vi "ziExample-HF2-QControl.vi"() -> ()   [LabVIEW 2009]
doc: "Control a Zurich instrument device via the LabOne Labview API. \nRequirements: Zurich Instruments HF2LI with HF2-MF and HF2-PID options.\nThis LabVIEW vi helps in configuring an HF2 to do Q-Control.\n\n© Zurich Instruments AG, www.zhinst.com"
uses:
  <instrlib>/Zurich Instruments LabOne/Public/Configure/ziSetValueDouble.vi
  <vilib>/Analysis/NI_AALPro.lvlib
  <vilib>/Utility/NIReport.llb/NI_report.lvclass
  <instrlib>/Zurich Instruments LabOne/Zurich Instruments LabOne.lvlib
panel:
  in  "restore settings":bool caption="Restore original settings"
  out "fmax":dbl=1000.0
  out "fmin":dbl=1000.0
  in  "Tab Control Sweep":enum32{"Sweeper", "Advanced Settings", "Help"}(tab)
  in  "Drive (V)":dbl=0.01 format="%.3g"
  out "Resonance Frequency Q":dbl
  in  "Run":bool caption="Run Sweep"
  out "Sweep Progress":dbl(slide) max=21.0 scale=0.0..1.0
  out "Graph Phase":T1(graph)=[{"Output (F,X1,Y1,X2,Y2,...,Vo)"=[1841839.1959798995, 1841849.2462311557, 1841859.2964824121, 1841869.3467336684, 1841879.3969849246, 1841889.447236181, 1841899.4974874372, 1841909.5477386934, 1841919.5979899496, 1841929.648241206, 1841939.6984924623, 1841949.7487437185, 1841959.798994975, 1841969.8492462311, 1841979.8994974873, 1841989.9497487438, 1842000.0, 1842010.0502512562, 1842020.1005025127, 1842030.1507537689, 1842040.201005025, 1842050.2512562815, 1842060.3015075377, 1842070.351758794, 1842080.4020100501, 1842090.4522613066, 1842100.5025125628, 1842110.552763819, 1842120.6030150754, 1842130.6532663316, 1842140.7035175879, 1842150.7537688443, 1842160.8040201005, 1842170.8542713567, 1842180.9045226132, 1842190.9547738694, 1842201.0050251256, 1842211.055276382, 1842221.1055276382, 1842231.1557788944, 1842241.2060301506, 1842251.256281407, 1842261.3065326633, 1842271.3567839195, 1842281.407035176, 1842291.4572864322, 1842301.5075376884, 1842311.5577889448, 1842321.608040201, 1842331.6582914572, 1842341.7085427137, 1842351.7587939699, 1842361.809045226, 1842371.8592964825, 1842381.9095477387, 1842391.959798995, 1842402.0100502511, 1842412.0603015076, 1842422.1105527638, 1842432.16080402, 1842442.2110552764, 1842452.2613065327, 1842462.3115577889, 1842472.3618090453, 1842482.4120603015, 1842492.4623115577, 1842502.5125628142, 1842512.5628140704, 1842522.6130653266, 1842532.6633165828, 1842542.7135678392, 1842552.7638190954, 1842562.8140703517, 1842572.864321608, 1842582.9145728643, 1842592.9648241205, 1842603.015075377, 1842613.0653266332, 1842623.1155778894, 1842633.1658291458, 1842643.216080402, 1842653.2663316582, 1842663.3165829147, 1842673.3668341709, 1842683.417085427, 1842693.4673366833, 1842703.5175879397, 1842713.567839196, 1842723.6180904522, 1842733.6683417086, 1842743.7185929648, 1842753.768844221, 1842763.8190954775, 1842773.8693467337, 1842783.9195979899, 1842793.9698492463, 1842804.0201005025, 1842814.0703517587, 1842824.1206030152, 1842834.1708542714, 1842844.2211055276, 1842854.2713567838, 1842864.3216080402, 1842874.3718592965, 1842884.4221105527, 1842894.472361809, 1842904.5226130653, 1842914.5728643215, 1842924.623115578, 1842934.6733668342, 1842944.7236180904, 1842954.7738693468, 1842964.824120603, 1842974.8743718592, 1842984.9246231157, 1842994.974874372, 1843005.025125628, 1843015.0753768843, 1843025.1256281408, 1843035.175879397, 1843045.2261306532, 1843055.2763819096, 1843065.3266331658, 1843075.376884422, 1843085.4271356785, 1843095.4773869347, 1843105.527638191, 1843115.5778894473, 1843125.6281407035, 1843135.6783919598, 1843145.7286432162, 1843155.7788944724, 1843165.8291457286, 1843175.8793969848, 1843185.9296482413, 1843195.9798994975, 1843206.0301507537, 1843216.0804020101, 1843226.1306532663, 1843236.1809045225, 1843246.231155779, 1843256.2814070352, 1843266.3316582914, 1843276.3819095478, 1843286.432160804, 1843296.4824120603, 1843306.5326633165, 1843316.582914573, 1843326.6331658291, 1843336.6834170853, 1843346.7336683418, 1843356.783919598, 1843366.8341708542, 1843376.8844221106, 1843386.9346733668, 1843396.984924623, 1843407.0351758795, 1843417.0854271357, 1843427.135678392, 1843437.1859296483, 1843447.2361809046, 1843457.2864321608, 1843467.336683417, 1843477.3869346734, 1843487.4371859296, 1843497.4874371858, 1843507.5376884423, 1843517.5879396985, 1843527.6381909547, 1843537.6884422111, 1843547.7386934673, 1843557.7889447236, 1843567.83919598, 1843577.8894472362, 1843587.9396984924, 1843597.9899497489, 1843608.040201005, 1843618.0904522613, 1843628.1407035175, 1843638.190954774, 1843648.2412060301, 1843658.2914572863, 1843668.3417085428, 1843678.391959799, 1843688.4422110552, 1843698.4924623116, 1843708.5427135678, 1843718.592964824, 1843728.6432160805, 1843738.6934673367, 1843748.743718593, 1843758.7939698494, 1843768.8442211056, 1843778.8944723618, 1843788.944723618, 1843798.9949748744, 1843809.0452261306, 1843819.0954773868, 1843829.1457286433, 1843839.1959798995], "dX/dt"=[-6.94293659208085, -7.039263365714603, -7.015747865746605, -7.022831577183382, -7.070140649231355, -7.097687461922305, -7.105617775743133, -7.187018771027357, -7.215555605807255, -7.209120372797453, -7.222963353111247, -7.2482145424437725, -7.336471988299522, -7.392871009974112, -7.404378015656745, -7.392520359287413, -7.520355608686046, -7.519542598388936, -7.550628880706965, -7.581504623203495, -7.613602056591421, -7.5885724211422065, -7.700014320037284, -7.728140979121345, -7.810709171761543, -7.784263466588973, -7.881518062030821, -7.903674328964446, -7.971719351332499, -8.017529667992314, -8.058121436672986, -8.165785698106287, -8.19016022550502, -8.212700433959935, -8.32675261509468, -8.371215456694097, -8.455244319826404, -8.452589972505562, -8.593897328803308, -8.603598584374405, -8.66788383890823, -8.728838589412112, -8.92008246055265, -8.96248928060953, -9.014325061381626, -9.12099819745259, -9.192260387685824, -9.25577287991073, -9.393754573052911, -9.510460418962696, -9.588798588744128, -9.671919305255168, -9.807909390069907, -9.872318951901494, -10.029523543826793, -10.111178612582068, -10.282365199143047, -10.41392827403316, -10.600908552099941, -10.721664299953895, -10.861537419641733, -11.05386683133099, -11.226967260541015, -11.399833261360014, -11.614266576451872, -11.822489241822097, -12.037591738878548, -12.284275795570396, -12.537696676929697, -12.808591866080967, -13.10897592112657, -13.414554360121997, -13.74678013981217, -14.102456694459267, -14.476936500710565, -14.894674114827959, -15.339877668460199, -15.812096714688613, -16.374409982820275, -16.9513079644051, -17.5854888581396, -18.28427561683263, -19.054069906143813, -19.928879874410452, -20.90995289279427, -21.975478569369823, -23.22079284159497, -24.61324931082536, -26.23607602255107, -28.12290317293296, -30.316540859101774, -32.93351414204068, -36.0685114581311, -39.86225308894581, -44.52062048412513, -50.265070638918324, -57.397192144852305, -66.16528396414377, -76.63221848917898, -88.4706687072364, -100.82403856696656, -112.6132379050097, -122.9993546962758, -131.68277440223207, -138.73027439508525, -144.42272136521782, -149.00962859772702, -152.74574201067415, -155.83478009073983, -158.4057569715815, -160.55712878950192, -162.41389955531858, -163.98916270213934, -165.35435338829546, -166.5502332885727, -167.6188034018421, -168.54149862098475, -169.38780172777604, -170.13679818450444, -170.78748418559624, -171.41172295788104, -171.99098890699028, -172.50066268325997, -172.9556325234782, -173.4008952713357, -173.82760697801268, -174.17343776744914, -174.55598606411053, -174.82677313412782, -175.20114654856826, -175.44438260372488, -175.74183048219098, -176.00347473058068, -176.23123546164112, -176.43388652935894, -176.62506543519825, -176.8656495868036, -177.000286426292, -177.2712077683475, -177.36028159834026, -177.53319063513797, -177.67555828450963, -177.84294696805748, -178.0118748631806, -178.16232009535963, -178.27551219372313, -178.39423075255817, -178.4903282214428, -178.5715733424731, -178.73836280736876, -178.82943056728186, -178.9850843467714, -179.04192894715334, -179.08270482893664, -179.19287748311572, -179.28322843883868, -179.34165759880761, -179.50709018669053, -179.4954309299658, -179.64736857972363, -179.60928252514617, -179.78420449956272, -179.8065606796536, -179.84218357544378, -179.90164268987297, -179.9062773498495, -180.0402030141334, -180.21011520251875, -180.02003421747088, -180.17501517626974, -180.197905755971, -180.35296807746022, -180.37609298337136, -180.54331181359302, -180.49811587577673, -180.50365280444166, -180.6359768081795, -180.47976323601006, -180.5713600449198, -180.67329316815656, -180.6154046528325, -180.75094639042254, -180.5940820677559, -180.83667931766678, -180.72000977161738, -180.90668274161465, -180.88415063790313, -180.91032933351386, -180.93791455694205, -180.8862600292335, -180.9706632041318, -181.0058055371726, -181.12385131631882, -180.99226180353708, -181.17117500602515, -181.20440954183448, -181.1560016539221, -181.11269108982725, -181.29568987605847, -181.260867961045]}, {"Output (F,X1,Y1,X2,Y2,...,Vo)"=array[500 elements], "dX/dt"=array[500 elements]}] caption="Graph2"
  out "Graph Amplitude":T2(graph)=[{"Output (F,X1,Y1,X2,Y2,...,Vo)"=[1841839.1959798995, 1841849.2462311557, 1841859.2964824121, 1841869.3467336684, 1841879.3969849246, 1841889.447236181, 1841899.4974874372, 1841909.5477386934, 1841919.5979899496, 1841929.648241206, 1841939.6984924623, 1841949.7487437185, 1841959.798994975, 1841969.8492462311, 1841979.8994974873, 1841989.9497487438, 1842000.0, 1842010.0502512562, 1842020.1005025127, 1842030.1507537689, 1842040.201005025, 1842050.2512562815, 1842060.3015075377, 1842070.351758794, 1842080.4020100501, 1842090.4522613066, 1842100.5025125628, 1842110.552763819, 1842120.6030150754, 1842130.6532663316, 1842140.7035175879, 1842150.7537688443, 1842160.8040201005, 1842170.8542713567, 1842180.9045226132, 1842190.9547738694, 1842201.0050251256, 1842211.055276382, 1842221.1055276382, 1842231.1557788944, 1842241.2060301506, 1842251.256281407, 1842261.3065326633, 1842271.3567839195, 1842281.407035176, 1842291.4572864322, 1842301.5075376884, 1842311.5577889448, 1842321.608040201, 1842331.6582914572, 1842341.7085427137, 1842351.7587939699, 1842361.809045226, 1842371.8592964825, 1842381.9095477387, 1842391.959798995, 1842402.0100502511, 1842412.0603015076, 1842422.1105527638, 1842432.16080402, 1842442.2110552764, 1842452.2613065327, 1842462.3115577889, 1842472.3618090453, 1842482.4120603015, 1842492.4623115577, 1842502.5125628142, 1842512.5628140704, 1842522.6130653266, 1842532.6633165828, 1842542.7135678392, 1842552.7638190954, 1842562.8140703517, 1842572.864321608, 1842582.9145728643, 1842592.9648241205, 1842603.015075377, 1842613.0653266332, 1842623.1155778894, 1842633.1658291458, 1842643.216080402, 1842653.2663316582, 1842663.3165829147, 1842673.3668341709, 1842683.417085427, 1842693.4673366833, 1842703.5175879397, 1842713.567839196, 1842723.6180904522, 1842733.6683417086, 1842743.7185929648, 1842753.768844221, 1842763.8190954775, 1842773.8693467337, 1842783.9195979899, 1842793.9698492463, 1842804.0201005025, 1842814.0703517587, 1842824.1206030152, 1842834.1708542714, 1842844.2211055276, 1842854.2713567838, 1842864.3216080402, 1842874.3718592965, 1842884.4221105527, 1842894.472361809, 1842904.5226130653, 1842914.5728643215, 1842924.623115578, 1842934.6733668342, 1842944.7236180904, 1842954.7738693468, 1842964.824120603, 1842974.8743718592, 1842984.9246231157, 1842994.974874372, 1843005.025125628, 1843015.0753768843, 1843025.1256281408, 1843035.175879397, 1843045.2261306532, 1843055.2763819096, 1843065.3266331658, 1843075.376884422, 1843085.4271356785, 1843095.4773869347, 1843105.527638191, 1843115.5778894473, 1843125.6281407035, 1843135.6783919598, 1843145.7286432162, 1843155.7788944724, 1843165.8291457286, 1843175.8793969848, 1843185.9296482413, 1843195.9798994975, 1843206.0301507537, 1843216.0804020101, 1843226.1306532663, 1843236.1809045225, 1843246.231155779, 1843256.2814070352, 1843266.3316582914, 1843276.3819095478, 1843286.432160804, 1843296.4824120603, 1843306.5326633165, 1843316.582914573, 1843326.6331658291, 1843336.6834170853, 1843346.7336683418, 1843356.783919598, 1843366.8341708542, 1843376.8844221106, 1843386.9346733668, 1843396.984924623, 1843407.0351758795, 1843417.0854271357, 1843427.135678392, 1843437.1859296483, 1843447.2361809046, 1843457.2864321608, 1843467.336683417, 1843477.3869346734, 1843487.4371859296, 1843497.4874371858, 1843507.5376884423, 1843517.5879396985, 1843527.6381909547, 1843537.6884422111, 1843547.7386934673, 1843557.7889447236, 1843567.83919598, 1843577.8894472362, 1843587.9396984924, 1843597.9899497489, 1843608.040201005, 1843618.0904522613, 1843628.1407035175, 1843638.190954774, 1843648.2412060301, 1843658.2914572863, 1843668.3417085428, 1843678.391959799, 1843688.4422110552, 1843698.4924623116, 1843708.5427135678, 1843718.592964824, 1843728.6432160805, 1843738.6934673367, 1843748.743718593, 1843758.7939698494, 1843768.8442211056, 1843778.8944723618, 1843788.944723618, 1843798.9949748744, 1843809.0452261306, 1843819.0954773868, 1843829.1457286433, 1843839.1959798995], [-28.966250862681054, -28.908176655273337, -28.864467111398284, -28.808136126619875, -28.754602779877295, -28.681537195962324, -28.60547886691201, -28.542769551012277, -28.47986278834069, -28.413059310021236, -28.35033543586046, -28.29138537216195, -28.227086468764178, -28.15168084424244, -28.083132309459675, -28.006652538062877, -27.923391524657678, -27.862916544212467, -27.784208516740375, -27.70412391696607, -27.636354468592554, -27.55133643843743, -27.46146332129707, -27.389341692048106, -27.294868081757663, -27.219310281261595, -27.123230188479226, -27.03474855024407, -26.950586594813416, -26.85355121081612, -26.765683710166535, -26.675242143760556, -26.564063048008382, -26.474632733618588, -26.37565770196402, -26.280112494285053, -26.172991235949205, -26.072598624000236, -25.959534728054443, -25.860640493819343, -25.7465174301761, -25.631539306182212, -25.498858352667277, -25.39010824649092, -25.25774799718558, -25.142249321882026, -25.00555406360646, -24.887022970441244, -24.75211169976204, -24.617521743246748, -24.48274082231197, -24.3428232828688, -24.196009592241655, -24.047554642475653, -23.889297411413008, -23.739575356461376, -23.570294117173674, -23.41322125110465, -23.224954797726845, -23.058866498583328, -22.88382952274905, -22.69856576681898, -22.50867999213655, -22.31450162319383, -22.111370069423263, -21.90338344600061, -21.68504571797671, -21.461764169109074, -21.226543135169543, -20.99229287484784, -20.741801499413626, -20.479366183700762, -20.21176825406491, -19.937742640458776, -19.648956986305464, -19.3468251889951, -19.033496520395904, -18.701812675964042, -18.355682042916765, -17.99270040419432, -17.615604660651464, -17.21865908953786, -16.797539016940565, -16.356977304926286, -15.888200014085553, -15.391846986851675, -14.866834628179921, -14.309077261379437, -13.711689066706123, -13.074653632558586, -12.392712546398329, -11.663574717432795, -10.884371326060215, -10.054211061904741, -9.183959621011658, -8.284378130216394, -7.3946969716815065, -6.579866401883259, -5.946660172340811, -5.612275426625389, -5.660939792976745, -6.092597885403304, -6.819063594921346, -7.720596881253953, -8.692845639671399, -9.676601274917646, -10.63194093311314, -11.542743236475578, -12.406298891129273, -13.216035317601213, -13.98028024462563, -14.699677218013587, -15.379521411615144, -16.023339805333272, -16.632012788033276, -17.212135663274463, -17.763951487592156, -18.287404341430125, -18.79046016208909, -19.273915407845625, -19.736440474832023, -20.179725827914766, -20.608959575656495, -21.018134587427294, -21.422995318238737, -21.807627924716133, -22.17859768043806, -22.532821774822636, -22.88528270717979, -23.228299264102954, -23.55688511871147, -23.881717376684854, -24.19613894993444, -24.49895105674716, -24.802029226261308, -25.099837529936202, -25.392446478391577, -25.673862567600672, -25.947515476929528, -26.22420324643256, -26.473552872567087, -26.742550094460967, -27.00104527827544, -27.248345780939687, -27.491641603363373, -27.74480782051559, -27.98078562862448, -28.223226877341677, -28.4458543248418, -28.668372965623256, -28.91316733771661, -29.134686427564475, -29.34772484111448, -29.55621510607997, -29.784051895982245, -30.00136613401197, -30.219876575206612, -30.42218292074636, -30.618607334447535, -30.831568097485093, -31.031377814888664, -31.230073398030804, -31.42672173766795, -31.62404980158688, -31.819935098980814, -32.01368910890594, -32.20561075361435, -32.396695113595065, -32.58604024745495, -32.754436974363834, -32.96100063832588, -33.124166975360936, -33.323942883117475, -33.50090098141094, -33.683801355462585, -33.87460045378752, -34.03049976000201, -34.25189149349637, -34.40356326157614, -34.580744989166725, -34.75748170316221, -34.94748867729741, -35.11731073350964, -35.288783018518025, -35.44821022332193, -35.6213094778834, -35.8056140321162, -35.95929649243196, -36.124591783023774, -36.30593369611333, -36.503240497902596, -36.64816967067446, -36.79128348867193, -36.99164183710858, -37.143384953777364, -37.26823219562254, -37.49034966949507, -37.662154614518144, -37.81959794162762, -38.00695446481112]}, {"Output (F,X1,Y1,X2,Y2,...,Vo)"=array[500 elements], array[500 elements]}] caption="Graph1"
  out "Q Factor":dbl format="%_4f"
  out "Resonance Freq (Hz)":dbl
  out "Phase Shift (°)":dbl format="%#.2f"
  out "controlled":dbl format="%_4f"
  out "Gain Margin (dB)":dbl caption="native" format="%.2f"
  out "f/2Q (Hz)":dbl
  out "Characteristic Frequency Q":dbl
  in  "Output Demod":i32(ring)=6 items=["1", "2", "3", "4", "5", "6", "7", "8"]
  in  "Input Demod":i32(ring)=3 items=["1", "2", "3", "4", "5", "6"]
  in  "Steps":dbl=200.0
  in  "BW (Hz)":dbl=100.0
  in  "AutoBW":bool caption="Auto"
  in  "Sweep Oscillator":i32(ring) caption="Oscillator" items=["1", "2", "3", "4", "5", "6"]
  in  "Show Derivative and Filter":bool caption="Show demodulator filter and phase derivative in graphs"
  in  "Tab Control QControl":T3(tab)
  in  "PID Drive Limit (V)":dbl=10.0 format="%.3g"
  in  "Center Frequency (Hz)":dbl=1000000.0
  in  "Bandwidth (Hz)":dbl=1000.0
  in  "Q Control":bool caption="Enable"
  in  "HW Channel":i32(ring) caption="Hardware Channel" items=["1", "2"]
  in  "Q Enhancement":dbl(slide) scale=0.1..100.0
  in  "AutoCenter":bool caption="Auto Center"
  in  "PIDs":i32(ring) items=["1 and 2", "3 and 4"]
  in  "Oscillator":i32(ring)=2 items=["1", "2", "3", "4", "5", "6"]
  in  "Feedback Phase (deg)":dbl(slide) scale=-180.0..180.0
  in  "Feedback Gain (V/Vrms)":dbl(slide) scale=0.01..100.0
  in  "Invert Gain":bool caption="Invert"
  out "Stability Warning":bool
  in  "AutoPhase":bool caption="Auto"
  in  "Auto Gain":bool caption="Auto"
  out "ADC Over":bool
  in  "stop":bool
  # "Tested on: HF2LI+PID"
  # "Requires HF2LI with installed\nHF2-MF and HF2-PID options."
  # "Beta user help:\n1) Hook up the resonator to either HF in/out 1 or HF in/out 2\n\n2) Find out the approximate resonator resonance frequency and enter it to the field \"Center Frequency\"\n\n3) Specify \"Bandwidth\" to be about 5x the width of the resonance peak (*).\n\n4) Start a sweep to find the native (natural) behavior of the resonator. The exact resonance frequency, Q-factor, characteristic frequency, phase at resonance and gain margin will be extracted. These values are crucial for a proper Q enhancement. (**)\n\n5) Set the \"Q Enhancement\" slider to the desired balue (2 increases Q by a factor of two) and enable Q control.\n\n6) Start another sweep and compare the transfer functions.\n\n* Keep in mind that the resonance may not shift more than the Q-control bandwidth. Bandwidth should not be set to a higher value than 10kHz as the PID controllers can update the drive with about 100kHz.\n** The time constant setting for the sweeper should suit the characteristic frequency of the cantilever."
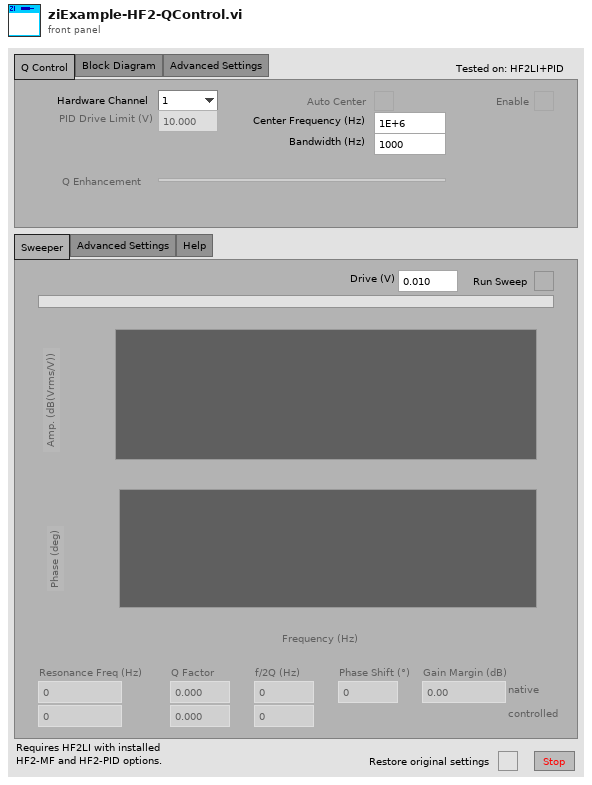
[diagram p1: front panel]
types:
  T1 = cluster{"Output (F,X1,Y1,X2,Y2,...,Vo)":dbl[], "dX/dt":dbl[]}[]
  T2 = cluster{"Output (F,X1,Y1,X2,Y2,...,Vo)":dbl[], dbl[]}[]
  T3 = enum32{"Q Control", "Block Diagram", "Advanced Settings"}
  T4 = typedef "Zurich Instruments LabOne.lvlib/ziTypeHandle.ctl" = cluster{"handleValid":bool, "Conn":u64, "Path Prefix":string, "Handle":u64, "Connected":bool, "Clockbase(s)":dbl}
  T5 = enum32{"Page Enabled", "Page Disabled", "Page Disabled & Grayed"}
  T6 = enum8{"Enabled", "Disabled", "Disabled and Grayed Out"}
  T7 = enum16{"Standard Report", "HTML", "Word", "Excel"}
  T8 = cluster{"Output (F,X1,Y1,X2,Y2,...,Vo)":dbl[], dbl[]}
  T9 = cluster{"Output (F,X1,Y1,X2,Y2,...,Vo)":dbl[], "Unwrapped Phase":dbl[]}
  T10 = enum32{"invalid app kind", "Development System", "Run Time System", "Student Edition", "Embedded LabVIEW", "Evaluation", "Custom"}
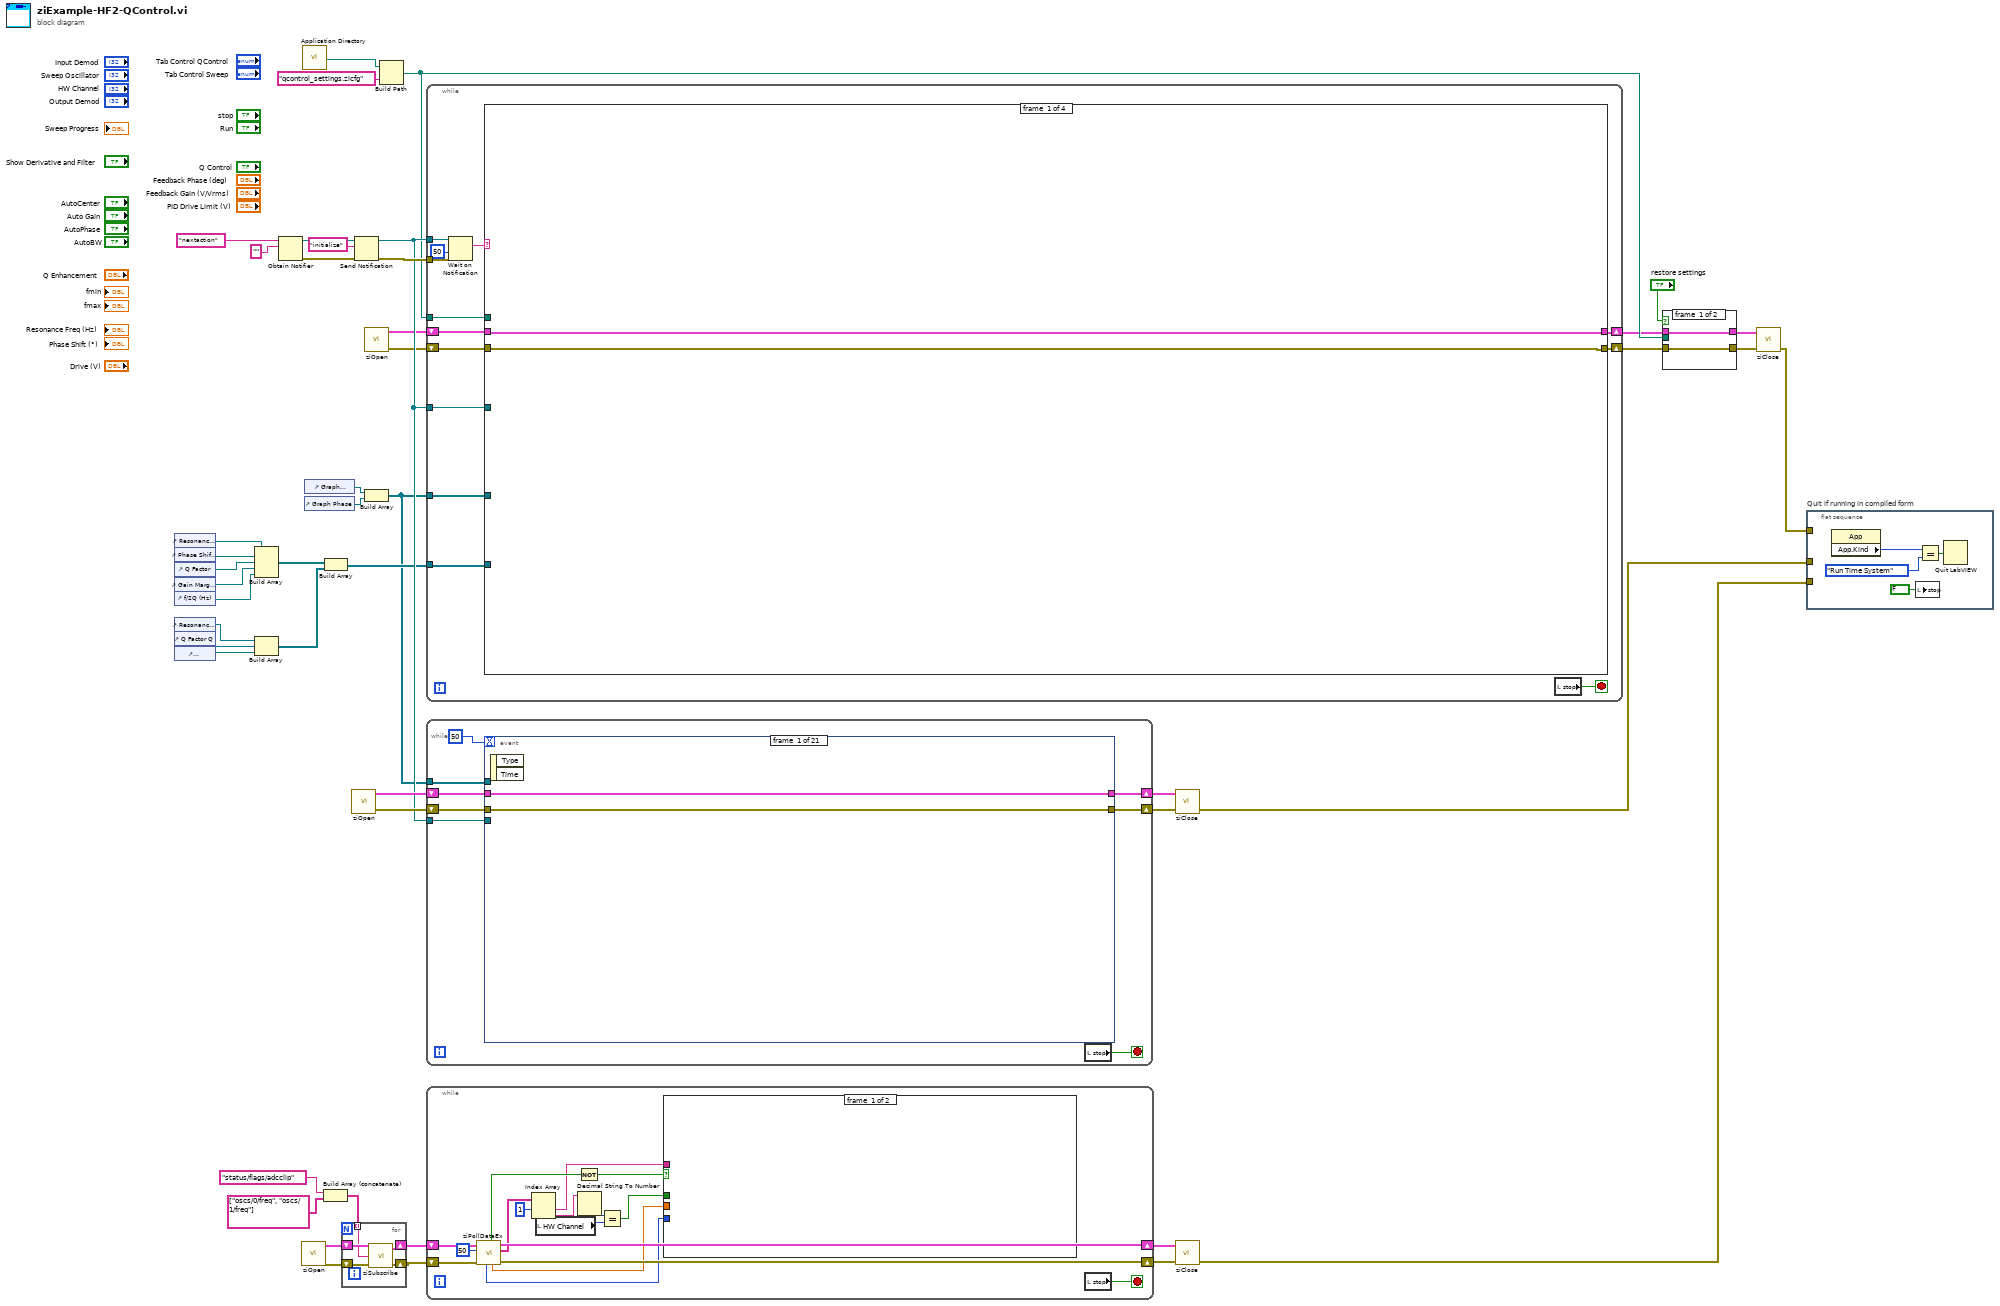
[diagram p0: block diagram]
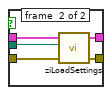
[diagram p2: hidden frame]
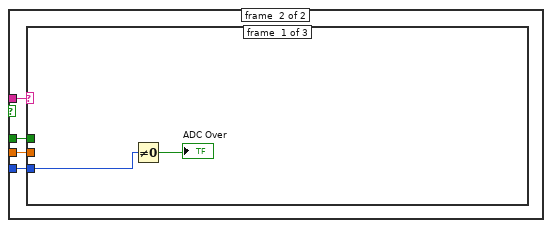
[diagram p3: hidden frame]
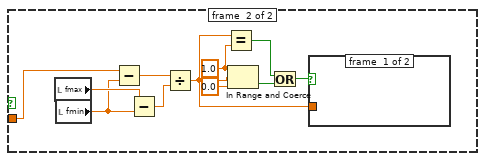
[diagram p6: hidden frame]
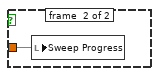
[diagram p7: hidden frame]
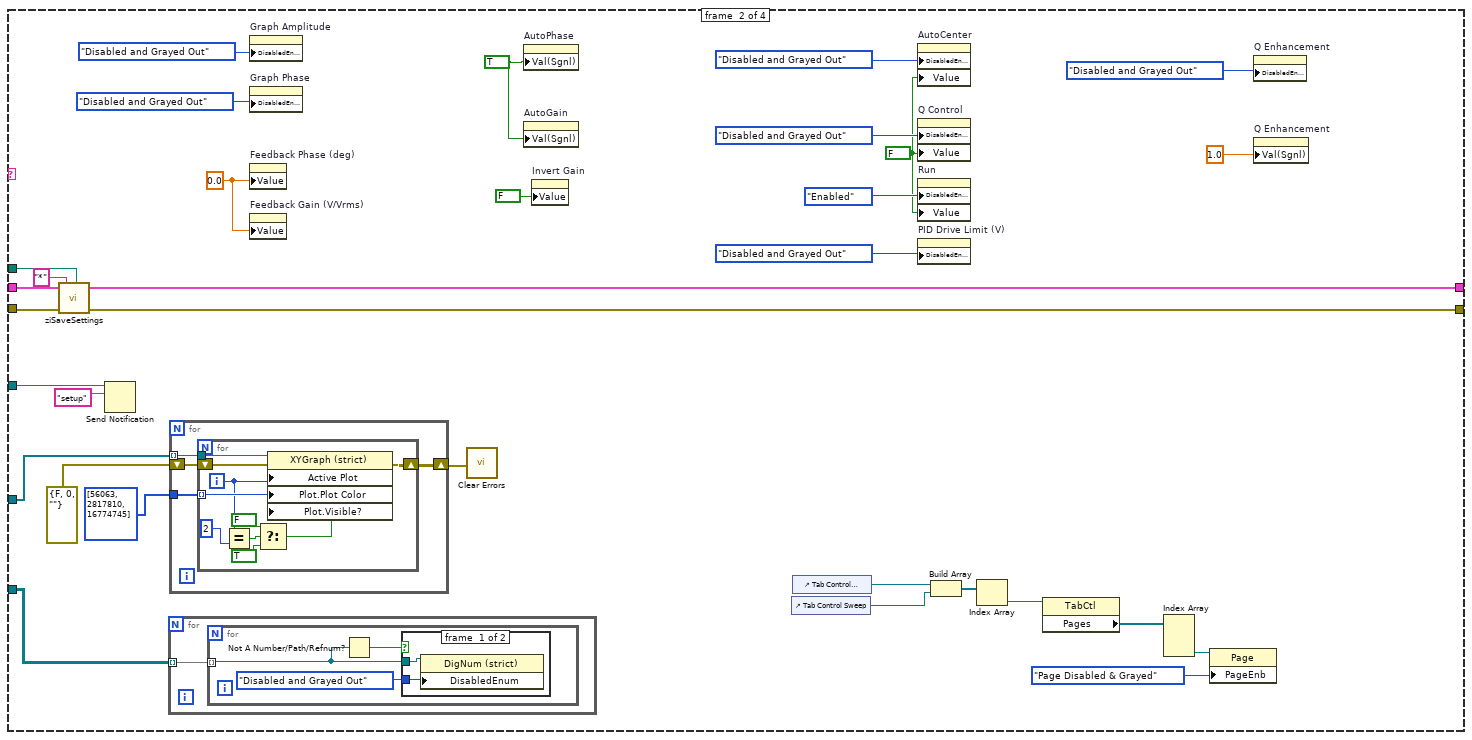
[diagram p8: hidden frame]
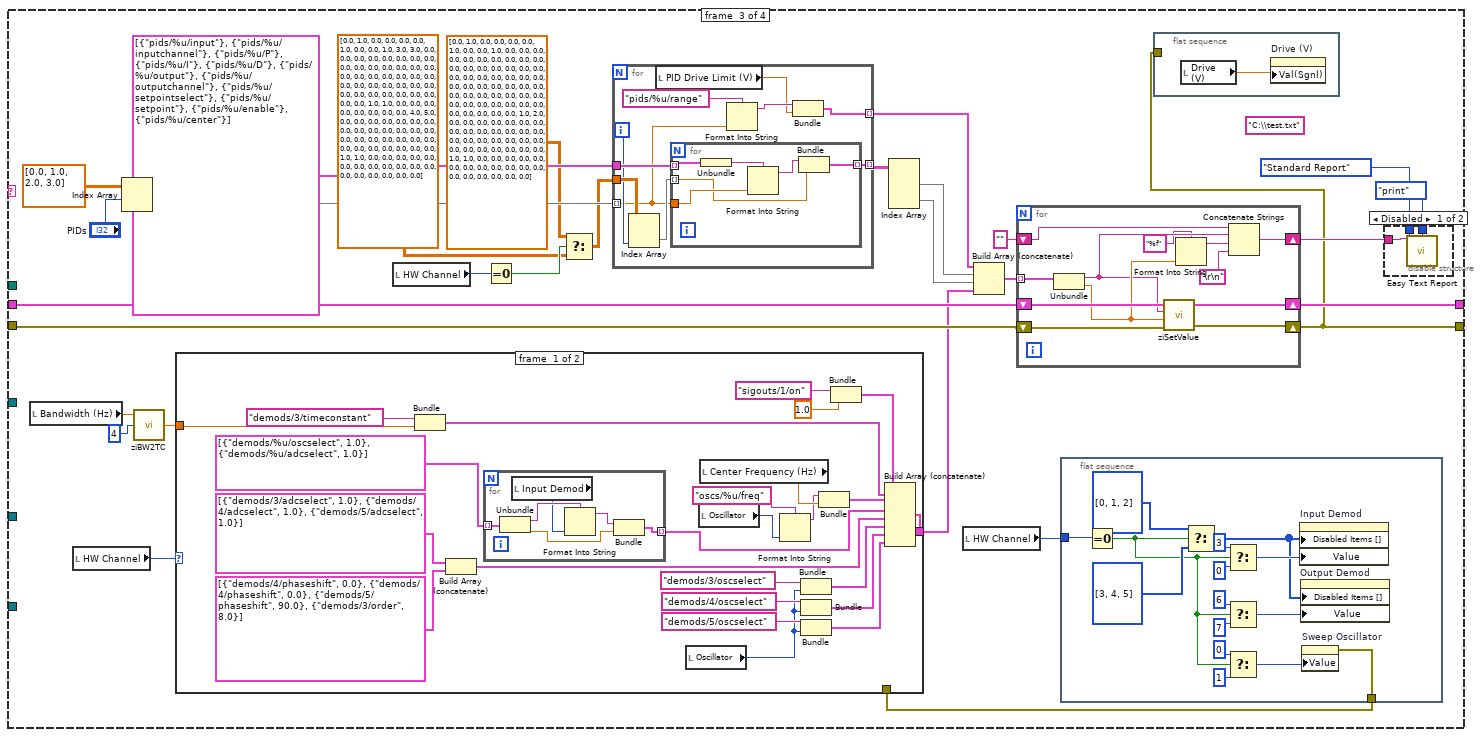
[diagram p10: hidden frame]
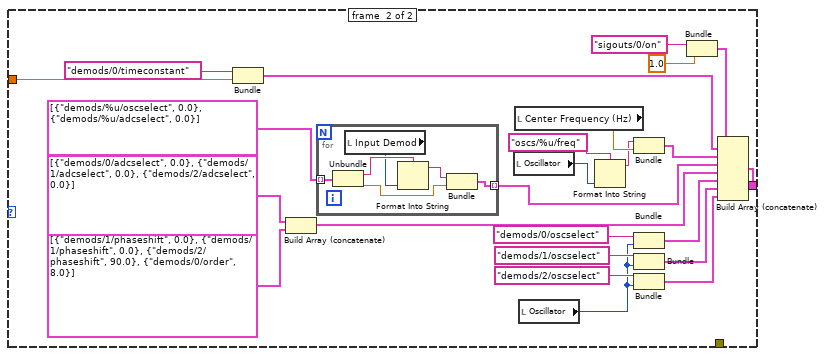
[diagram p12: hidden frame]
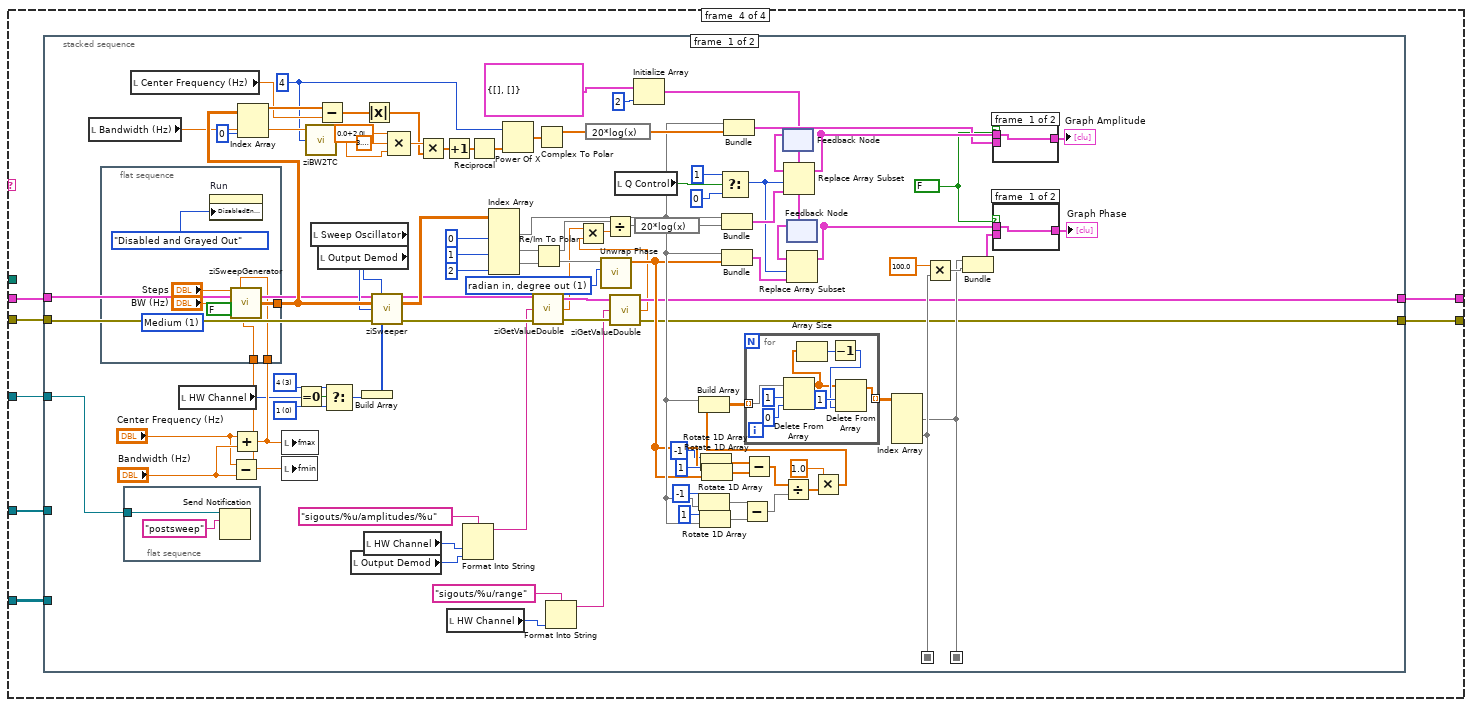
[diagram p13: hidden frame]
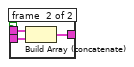
[diagram p14: hidden frame]
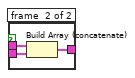
[diagram p15: hidden frame]
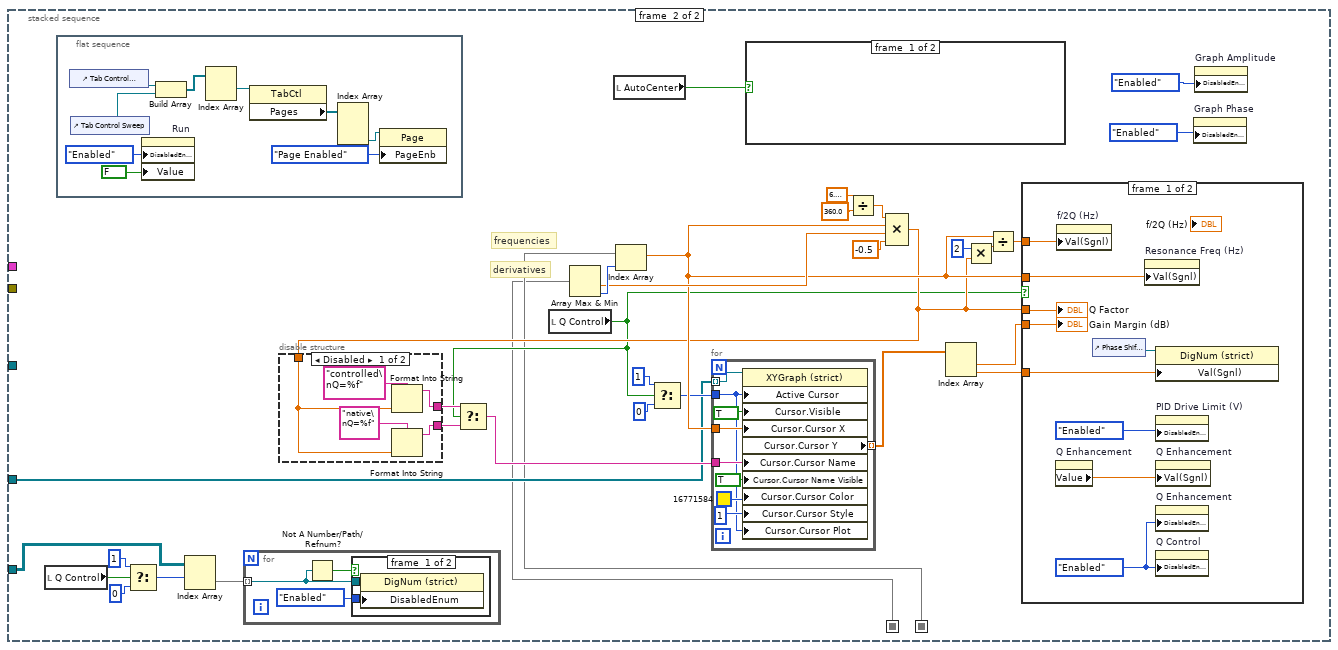
[diagram p16: hidden frame]
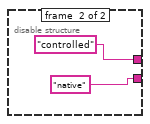
[diagram p17: hidden frame]
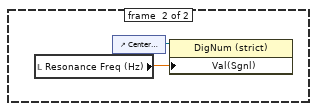
[diagram p18: hidden frame]
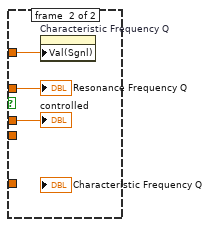
[diagram p20: hidden frame]
diagram:
  n1 = control-ref of="Resonance Freq (Hz)"() -> (w32:refnum<vi>)
  n2 = control-ref of="Phase Shift (°)"() -> (w31:refnum<vi>)
  n3 = control-ref of="Q Factor"() -> (w30:refnum<vi>)
  n4 = control-ref of="Gain Margin (dB)"() -> (w29:refnum<vi>)
  n5 = control-ref of="f/2Q (Hz)"() -> (w20:refnum<vi>)
  n6 = control-ref of="Resonance Frequency Q"() -> (w18:refnum<vi>)
  n7 = control-ref of="Q Factor Q"() -> (w28:refnum<vi>)
  n8 = control-ref of="Characteristic Frequency Q"() -> (w19:refnum<vi>)
  n9 = Build Array(w32, w31, w30, w29, w20) -> (w26:refnum<vi>[])
  n10 = Build Array(w18, w28, w19) -> (w27:refnum<vi>[])
  n11 = Obtain Notifier(name (unnamed)="nextaction", notification data type="") -> (notifier out=w45:refnum<notifier>, error out=w43:errorcluster)  [unwired: 2 in, 1 out]
  n12 = call <instrlib>:"ziOpen.vi"() -> ("Error Out"=w33:errorcluster, "HandleOut"=w34:T4)  [unwired: 4 in, 1 out]
  n13 = call <vilib>:"Application Directory.vi"() -> ("Application Directory"=w17:path)
  n14 = control-ref of="Graph Phase"() -> (w21:refnum<vi>)
  n15 = control-ref of="Graph Amplitude"() -> (w22:refnum<vi>)
  n16 = Build Array (concatenate)("status/flags/adcclip" ("Path ()"), string[] ["oscs/0/freq", "oscs/1/freq"]) -> (w7:string[])
  n17 = Build Array(w26, w27) -> (w25:refnum<vi>[][])
  n18 = for {
    tunnel: w7 -> [w48] mode=indexing
    shift-right: [w51] -> w5
    shift-left: w34 -> [w52]
    shift-right: [w50] -> w4
    shift-left: w33 -> [w49]
    n19 = call <instrlib>:"ziSubscribe.vi"("error in"=w49, "Path ()"=w48, "Handle In"=w52) -> ("error out"=w50:errorcluster, "Handle Out"=w51:T4)  [unwired: 1 in]
  }
  n20 = call <instrlib>:"ziOpen.vi"() -> ("Error Out"=w39:errorcluster, "HandleOut"=w41:T4)  [unwired: 4 in, 1 out]
  n21 = Send Notification(notification="initialize", notifier=w45, error in (no error)=w43) -> (notifier out=w37:refnum<notifier>, error out=w42:errorcluster)
  n22 = call <instrlib>:"ziOpen.vi"() -> ("Error Out"=w23:errorcluster, "HandleOut"=w24:T4)  [unwired: 4 in, 1 out]
  n23 = Build Array(w22, w21) -> (w9:refnum<vi>[])
  n24 = Build Path(base path=w17, name or relative path="qcontrol_settings.zicfg") -> (appended path=w15:path)
  n25 = while {
    tunnel: w37 -> [w64]
    tunnel: w42 -> [w62]
    tunnel: w37 -> [w60]
    tunnel: w25 -> [w59]
    shift-right: [w55] -> w14
    shift-left: w24 -> [w58]
    shift-right: [w56] -> w13
    shift-left: w23 -> [w57]
    tunnel: w9 -> [w54]
    tunnel: w15 -> [w53]
    stop <- w65 stop-if-true
    n26 = Wait on Notification(notifier=w64, timeout in ms (-1)=50, error in (no error)=w62) -> (notification=w63:string)  [unwired: 1 in, 3 out]
    n27 = case shown="\"setup\"" w63 {
      tunnel: w60 -> [_ w98 _ w257]
      tunnel: w59 -> [_ w96 _ w261]
      tunnel: w58 -> [w67 w86 w139 w260]
      tunnel: w57 -> [w66 w87 w138 w259]
      tunnel: [w66 w87 w120 w258] -> w56
      tunnel: [w67 w85 w137 w256] -> w55
      tunnel: w54 -> [_ w90 _ w255]
      tunnel: w53 -> [_ w83 _ _]
      frame #0 {
      }
      frame #1 {
        w82 = 0.0 ("Feedback Phase (deg)")
        w80 = TRUE ("AutoPhase")
        w88 = FALSE ("Q Control")
        n28 = call <instrlib>:"ziSaveSettings.vi"("Path (\"\")"="*" ("Path"), "file path (dialog if empty)"=w83, "Handle In"=w86) -> ("Handle Out"=w85:T4)  [unwired: 1 in, 2 out]
        n29 = Send Notification(notification="setup", notifier=w98) -> ()  [unwired: 1 in, 2 out]
        n30 = for {
          tunnel: w96 -> [w113] mode=indexing
          n31 = for {
            tunnel: w113 -> [w114] mode=indexing
            n32 = Not A Number/Path/Refnum?(number/path/refnum=w114) -> (NaN/Path/Refnum?=w115:bool)
            n33 = case shown="False" w115 {
              tunnel: T6."Disabled and Grayed Out" ("Disabled") -> [w118 _]
              tunnel: w114 -> [w117 _]
              frame #0 {
                n34 = property class="DigNum (strict)"(reference=w117, "DisabledEnum"=w118) -> ()  [unwired: 1 in, 2 out]
              }
              frame #1 {
              }
            }
          }
        }
        n35 = for {
          tunnel: w90 -> [w102] mode=indexing
          tunnel: u32[] [56063, 2817810, 16774745] -> [w101]
          shift-right: [w99] -> w91
          shift-left: errorcluster {"status"=FALSE, "code"=0, "source"=""} ("error in (no error)") -> [w100]
          n36 = for {
            tunnel: w102 -> [w112]
            tunnel: w101 -> [w111] mode=indexing
            shift-right: [w109] -> w99
            shift-left: w100 -> [w110]
            i -> [w108]
            n37 = Equal?(x=w108, y=2) -> (x = y?=w106:bool)
            n38 = Select(t=FALSE ("Plot.Visible"), s=w106, f=TRUE ("Plot.Visible")) -> (s? t:f=w105:bool)
            n39 = property class="XYGraph (strict)"(reference=w112, error in=w110, "Active Plot"=w108, "Plot.Plot Color"=w111, "Plot.Visible?"=w105) -> (error out=w109:errorcluster)  [unwired: 1 out]
          }
        }
        n40 = property on="Graph Amplitude" class="XYGraph (strict)"("DisabledEnum"=T6."Disabled and Grayed Out" ("Disabled")) -> ()  [unwired: 2 in, 2 out]
        n41 = property on="Graph Phase" class="XYGraph (strict)"("DisabledEnum"=T6."Disabled and Grayed Out" ("Disabled")) -> ()  [unwired: 2 in, 2 out]
        n42 = property on="Feedback Phase (deg)" class="Slide (strict)"("Value"=w82) -> ()  [unwired: 2 in, 2 out]
        n43 = property on="Feedback Gain (V/Vrms)" class="Slide (strict)"("Value"=w82) -> ()  [unwired: 2 in, 2 out]
        n44 = call <vilib>:"Clear Errors.vi"("error in (no error)"=w91) -> ()  [unwired: 6 in, 1 out]
        n45 = property on="AutoPhase" class="Bool (strict)"("Val(Sgnl)"=w80) -> ()  [unwired: 2 in, 2 out]
        n46 = property on="AutoGain" class="Bool (strict)"("Val(Sgnl)"=w80) -> ()  [unwired: 2 in, 2 out]
        n47 = property on="Invert Gain" class="Bool (strict)"("Value"=FALSE ("Invert Gain")) -> ()  [unwired: 2 in, 2 out]
        n48 = control-ref of="Tab Control Sweep"() -> (w78:refnum<vi>)
        n49 = control-ref of="Tab Control QControl"() -> (w79:refnum<vi>)
        n50 = property on="AutoCenter" class="Bool (strict)"("DisabledEnum"=T6."Disabled and Grayed Out" ("Disabled"), "Value"=w88) -> ()  [unwired: 2 in, 2 out]
        n51 = property on="Q Control" class="Bool (strict)"("DisabledEnum"=T6."Disabled and Grayed Out" ("Disabled"), "Value"=w88) -> ()  [unwired: 2 in, 2 out]
        n52 = property on="Run" class="Bool (strict)"("DisabledEnum"=T6."Enabled" ("Disabled"), "Value"=w88) -> ()  [unwired: 2 in, 2 out]
        n53 = property on="PID Drive Limit (V)" class="DigNum (strict)"("DisabledEnum"=T6."Disabled and Grayed Out" ("Disabled")) -> ()  [unwired: 2 in, 2 out]
        n54 = Build Array(w79, w78) -> (w71:refnum<vi>[])
        n55 = Index Array(array=w71) -> (element=w70:refnum<vi>)  [unwired: 1 in]
        n56 = property class="TabCtl"(reference=w70) -> ("Pages"=w73:refnum<vi>[])  [unwired: 1 in, 2 out]
        n57 = Index Array(array=w73) -> (element #3=w69:refnum<vi>)  [unwired: 3 in, 2 out]
        n58 = property class="Page"(reference=w69, "PageEnb"=T5."Page Disabled & Grayed" ("Page Enabled State")) -> ()  [unwired: 1 in, 2 out]
        n59 = property on="Q Enhancement" class="Slide (strict)"("DisabledEnum"=T6."Disabled and Grayed Out" ("Disabled")) -> ()  [unwired: 2 in, 2 out]
        n60 = property on="Q Enhancement" class="Slide (strict)"("Val(Sgnl)"=1.0 ("Q Enhancement")) -> ()  [unwired: 2 in, 2 out]
      }
      frame #2 {
        (unwired) "C:\\test.txt" ("printer name (default) or file path (dialog)")
        n61 = local read "Bandwidth (Hz)"() -> (w147:dbl)
        n62 = local read "HW Channel"() -> (w144:i32)
        n63 = Index Array(array=dbl[][] [[0.0, 1.0], [2.0, 3.0]], index (row)="PIDs") -> (element=w141:dbl[])  [unwired: 1 in]
        n64 = call <instrlib>:"ziBW2TC.vi"("Order (1)"=4 ("Order (#)"), "BW (Hz)"=w147) -> ("TC (s)"=w145:dbl)  [unwired: 1 in]
        n65 = case shown="1" w144 {
          tunnel: [w215 w243] -> w136
          tunnel: w145 -> [w207 w235]
          tunnel: w119 -> [_ _]
          frame #0 {
            n66 = Bundle("demods/3/timeconstant", "TC (s)"=w207) -> (w206:cluster{string, "TC (s)":dbl})  [unwired: 1 in]
            n67 = Build Array (concatenate)(cluster{string, dbl}[] [{"demods/3/adcselect", 1.0}, {"demods/4/adcselect", 1.0}, {"demods/5/adcselect", 1.0}], cluster{string, dbl}[] [{"demods/4/phaseshift", 0.0}, {"demods/4/phaseshift", 0.0}, {"demods/5/phaseshift", 90.0}, {"demods/3/order", 8.0}]) -> (w203:cluster{string, dbl}[])
            n68 = for {
              tunnel: cluster{string, dbl}[] [{"demods/%u/oscselect", 1.0}, {"demods/%u/adcselect", 1.0}] -> [w224] mode=indexing
              tunnel: [w222] -> w210 mode=indexing
              n69 = Unbundle(w224) -> (w223:string, w220:dbl)
              n70 = local read "Input Demod"() -> (w219:i32)
              n71 = Format Into String(format string=w223, w219) -> (resulting string=w221:string)  [unwired: 2 in, 1 out]
              n72 = Bundle(w221, w220) -> (w222:cluster{string, dbl})  [unwired: 1 in]
            }
            n73 = local read "Oscillator"() -> (w211:i32)
            n74 = local read "Oscillator"() -> (w199:i32)
            n75 = local read "Center Frequency (Hz)"() -> (w202:dbl)
            n76 = Format Into String(format string="oscs/%u/freq", w199) -> (resulting string=w200:string)  [unwired: 2 in, 1 out]
            n77 = Bundle("demods/3/oscselect", "Oscillator"=w211) -> (w214:cluster{string, "Oscillator":i32})  [unwired: 1 in]
            n78 = Bundle("demods/4/oscselect", "Oscillator"=w211) -> (w213:cluster{string, "Oscillator":i32})  [unwired: 1 in]
            n79 = Bundle("demods/5/oscselect", "Oscillator"=w211) -> (w212:cluster{string, "Oscillator":i32})  [unwired: 1 in]
            n80 = Bundle(w200, "Center Frequency (Hz)"=w202) -> (w198:cluster{string, "Center Frequency (Hz)":dbl})  [unwired: 1 in]
            n81 = Bundle("sigouts/1/on", "TC (s)"=1.0) -> (w195:cluster{string, "TC (s)":dbl})  [unwired: 1 in]
            n82 = Build Array (concatenate)(w195, w206, w198, w210, w203, w214, w213, w212) -> (w215:cluster{string, "Center Frequency (Hz)":dbl}[])
          }
          frame #1 {
            n83 = Bundle("demods/0/timeconstant", "TC (s)"=w235) -> (w234:cluster{string, "TC (s)":dbl})  [unwired: 1 in]
            n84 = Build Array (concatenate)(cluster{string, dbl}[] [{"demods/0/adcselect", 0.0}, {"demods/1/adcselect", 0.0}, {"demods/2/adcselect", 0.0}], cluster{string, dbl}[] [{"demods/1/phaseshift", 0.0}, {"demods/1/phaseshift", 0.0}, {"demods/2/phaseshift", 90.0}, {"demods/0/order", 8.0}]) -> (w231:cluster{string, dbl}[])
            n85 = for {
              tunnel: cluster{string, dbl}[] [{"demods/%u/oscselect", 0.0}, {"demods/%u/adcselect", 0.0}] -> [w254] mode=indexing
              tunnel: [w252] -> w238 mode=indexing
              n86 = Unbundle(w254) -> (w253:string, w250:dbl)
              n87 = local read "Input Demod"() -> (w249:i32)
              n88 = Format Into String(format string=w253, w249) -> (resulting string=w251:string)  [unwired: 2 in, 1 out]
              n89 = Bundle(w251, w250) -> (w252:cluster{string, dbl})  [unwired: 1 in]
            }
            n90 = local read "Oscillator"() -> (w228:i32)
            n91 = local read "Center Frequency (Hz)"() -> (w247:dbl)
            n92 = local read "Oscillator"() -> (w239:i32)
            n93 = Format Into String(format string="oscs/%u/freq", w228) -> (resulting string=w229:string)  [unwired: 2 in, 1 out]
            n94 = Bundle(w229, "Center Frequency (Hz)"=w247) -> (w248:cluster{string, "Center Frequency (Hz)":dbl})  [unwired: 1 in]
            n95 = Bundle("demods/0/oscselect", "Oscillator"=w239) -> (w242:cluster{string, "Oscillator":i32})  [unwired: 1 in]
            n96 = Bundle("demods/1/oscselect", "Oscillator"=w239) -> (w241:cluster{string, "Oscillator":i32})  [unwired: 1 in]
            n97 = Bundle("demods/2/oscselect", "Oscillator"=w239) -> (w240:cluster{string, "Oscillator":i32})  [unwired: 1 in]
            n98 = Bundle("sigouts/0/on", "TC (s)"=1.0) -> (w225:cluster{string, "TC (s)":dbl})  [unwired: 1 in]
            n99 = Build Array (concatenate)(w225, w234, w248, w238, w231, w242, w241, w240) -> (w243:cluster{string, "Center Frequency (Hz)":dbl}[])
          }
        }
        n100 = local read "HW Channel"() -> (w127:i32)
        n101 = Equal To 0?(x=w127) -> (x = 0?=w126:bool)
        n102 = Select(t=dbl[][] [[0.0, 1.0, 0.0, 0.0, 0.0, 0.0, 1.0, 0.0, 0.0, 1.0], [0.0, 0.0, 0.0, 0.0, 0.0, 0.0, 0.0, 0.0, 0.0, 0.0], [0.0, 0.0, 0.0, 0.0, 0.0, 0.0, 0.0, 0.0, 0.0, 0.0], [0.0, 0.0, 0.0, 0.0, 0.0, 0.0, 0.0, 0.0, 0.0, 0.0], [0.0, 0.0, 0.0, 0.0, 0.0, 0.0, 0.0, 0.0, 0.0, 0.0], [0.0, 0.0, 0.0, 0.0, 0.0, 0.0, 0.0, 0.0, 0.0, 0.0], [1.0, 2.0, 0.0, 0.0, 0.0, 0.0, 0.0, 0.0, 0.0, 0.0], [0.0, 0.0, 0.0, 0.0, 0.0, 0.0, 0.0, 0.0, 0.0, 0.0], [0.0, 0.0, 0.0, 0.0, 0.0, 0.0, 0.0, 0.0, 0.0, 0.0], [1.0, 1.0, 0.0, 0.0, 0.0, 0.0, 0.0, 0.0, 0.0, 0.0], [0.0, 0.0, 0.0, 0.0, 0.0, 0.0, 0.0, 0.0, 0.0, 0.0]], s=w126, f=dbl[][] [[0.0, 1.0, 0.0, 0.0, 0.0, 0.0, 1.0, 0.0, 0.0, 1.0], [3.0, 3.0, 0.0, 0.0, 0.0, 0.0, 0.0, 0.0, 0.0, 0.0], [0.0, 0.0, 0.0, 0.0, 0.0, 0.0, 0.0, 0.0, 0.0, 0.0], [0.0, 0.0, 0.0, 0.0, 0.0, 0.0, 0.0, 0.0, 0.0, 0.0], [0.0, 0.0, 0.0, 0.0, 0.0, 0.0, 0.0, 0.0, 0.0, 0.0], [1.0, 1.0, 0.0, 0.0, 0.0, 0.0, 0.0, 0.0, 0.0, 0.0], [4.0, 5.0, 0.0, 0.0, 0.0, 0.0, 0.0, 0.0, 0.0, 0.0], [0.0, 0.0, 0.0, 0.0, 0.0, 0.0, 0.0, 0.0, 0.0, 0.0], [0.0, 0.0, 0.0, 0.0, 0.0, 0.0, 0.0, 0.0, 0.0, 0.0], [1.0, 1.0, 0.0, 0.0, 0.0, 0.0, 0.0, 0.0, 0.0, 0.0], [0.0, 0.0, 0.0, 0.0, 0.0, 0.0, 0.0, 0.0, 0.0, 0.0]]) -> (s? t:f=w123:dbl[][])
        n103 = for {
          tunnel: w141 -> [w179] mode=indexing
          tunnel: cluster{string}[] [{"pids/%u/input"}, {"pids/%u/inputchannel"}, {"pids/%u/P"}, {"pids/%u/I"}, {"pids/%u/D"}, {"pids/%u/output"}, {"pids/%u/outputchannel"}, {"pids/%u/setpointselect"}, {"pids/%u/setpoint"}, {"pids/%u/enable"}, {"pids/%u/center"}] -> [w188]
          tunnel: [w187] -> w134 mode=indexing
          tunnel: w123 -> [w186]
          tunnel: [w181] -> w121 mode=indexing
          i -> [w183]
          n104 = Index Array(array=w186, index (col)=w183) -> (element=w185:dbl[])  [unwired: 1 in]
          n105 = local read "PID Drive Limit (V)"() -> (w180:dbl)
          n106 = for {
            tunnel: w188 -> [w190] mode=indexing
            tunnel: w179 -> [w193]
            tunnel: [w192] -> w187 mode=indexing
            tunnel: w185 -> [w191] mode=indexing
            n107 = Unbundle(w190) -> (w189:string)
            n108 = Format Into String(format string=w189, w193) -> (resulting string=w194:string)  [unwired: 2 in, 1 out]
            n109 = Bundle(w194, w191) -> (w192:cluster{string, dbl})  [unwired: 1 in]
          }
          n110 = Format Into String(format string="pids/%u/range", w179) -> (resulting string=w182:string)  [unwired: 2 in, 1 out]
          n111 = Bundle(w182, "PID Drive Limit (V)"=w180) -> (w181:cluster{string, "PID Drive Limit (V)":dbl})  [unwired: 1 in]
        }
        n112 = Index Array(array=w134) -> (element #1=w133:cluster{string, dbl}[], element #2=w132:cluster{string, dbl}[])  [unwired: 4 in]
        n113 = local read "HW Channel"() -> (w122:i32)
        n114 = Build Array (concatenate)(w121, w133, w132, w136) -> (w135:cluster{string, "Center Frequency (Hz)":dbl}[])
        n115 = for {
          tunnel: w135 -> [w174] mode=indexing
          shift-right: [w177] -> w137
          shift-left: w139 -> [w178]
          shift-right: [w175] -> w120
          shift-left: w138 -> [w176]
          shift-right: [w170] -> w131
          shift-left: "" -> [w169]
          n116 = Unbundle(w174) -> (w171:string, "Center Frequency (Hz)"=w173:dbl)
          n117 = call-poly <instrlib>:"ziSetValue.vi"("Error In"=w176, "Value"=w173, "Path"=w171, "Handle In"=w178) -> ("Error Out"=w175:errorcluster, "Handle Out"=w177:T4)  [unwired: 1 in]
          n118 = Format Into String(format string="%f" ("initial string"), w173) -> (resulting string=w172:string)  [unwired: 2 in, 1 out]
          n119 = Concatenate Strings(w169, w171, w172, "\r\n") -> (w170:string)
        }
        n120 = flat-sequence {
          tunnel: w122 -> [w163]
          tunnel: [w149] -> w119
          frame #0 {
            n121 = Equal To 0?(x=w163) -> (x = 0?=w150:bool)
            n122 = Select(t=i32[] [0, 1, 2] ("Disabled Items []"), s=w150, f=i32[] [3, 4, 5] ("Disabled Items []")) -> (s? t:f=w157:i32[])
            n123 = Select(t=3, s=w150, f=0) -> (s? t:f=w160:i32)
            n124 = Select(t=6, s=w150, f=7) -> (s? t:f=w154:i32)
            n125 = Select(t=0, s=w150, f=1) -> (s? t:f=w151:i32)
            n126 = property on="Input Demod" class="Ring (strict)"("Disabled Items []"=w157, "Value"=w160) -> ()  [unwired: 2 in, 2 out]
            n127 = property on="Output Demod" class="Ring (strict)"("Disabled Items []"=w157, "Value"=w154) -> ()  [unwired: 2 in, 2 out]
            n128 = property on="Sweep Oscillator" class="Ring (strict)"("Value"=w151) -> (error out=w149:errorcluster)  [unwired: 2 in, 1 out]
          }
        }
        n129 = flat-sequence {
          tunnel: w120 -> [_]
          frame #0 {
            n130 = local read "Drive (V)"() -> (w148:dbl)
            n131 = property on="Drive (V)" class="DigNum (strict)"("Val(Sgnl)"=w148) -> ()  [unwired: 2 in, 2 out]
          }
        }
        n132 = disable-structure shown="Disabled" {
          disable-tunnel: w131 -> [w166 _]
          disable-tunnel: enum16{"print", "save"}."print" ("print or save? (Word/Excel/HTML)") -> [w165 _]
          disable-tunnel: T7."Standard Report" ("report type") -> [w164 _]
          frame #0 {
            n133 = call <vilib>:"Easy Text Report.vi"("text to be printed"=w166, "print or save? (Word/Excel/HTML)"=w165, "report type"=w164) -> ()  [unwired: 12 in, 1 out]
          }
          frame #1 {
          }
        }
      }
      frame #3 {
        n134 = stacked-sequence {
          seq-local: [w272 _] -> [_ w392]
          seq-local: [w273 _] -> [_ w391]
          tunnel: w261 -> [_ w390]
          tunnel: w260 -> [w285 _]
          tunnel: w259 -> [w284 _]
          tunnel: [w266 _] -> w258
          tunnel: w257 -> [w274 _]
          tunnel: [w268 _] -> w256
          tunnel: w255 -> [_ w397]
          frame #0 {
            w278 = 0 items=["1", "2", "3", "4", "5", "6"] ("Sweep Oscillator")
            w305 = FALSE
            w279 = 3 items=["1", "2", "3", "4", "5", "6"] ("Sweep Oscillator")
            w288 = 4 ("Order (#)")
            w351 = 1 items=["radian in, radian out", "radian in, degree out", "degree in, degree out", "degree in, radian out"] ("phase unit")
            n135 = local read "Bandwidth (Hz)"() -> (w331:dbl)
            n136 = flat-sequence {
              tunnel: [w384] -> w360
              tunnel: w280 -> [w380]
              tunnel: w281 -> [w379]
              frame #0 {
                w386 = 1 items=["Low", "Medium", "High"] ("Precision (Low)")
                n137 = property on="Run" class="Bool (strict)"("DisabledEnum"=T6."Disabled and Grayed Out" ("Disabled")) -> ()  [unwired: 2 in, 2 out]
                n138 = call <instrlib>:"ziSweepGenerator.vi"("Steps (#)"="Steps", "Start (Hz)"=w380, "Bandwith (-1=auto)"="BW (Hz)", "Log Sweep (true)"=FALSE, "Precision (Low)"=w386, "Stop (Hz)"=w379) -> ("Sweep Sequence (F (Hz), BW (Hz), TC(s), Time(s))"=w384:dbl[][])  [unwired: 7 in, 2 out]
              }
            }
            n139 = flat-sequence {
              tunnel: w274 -> [w361]
              frame #0 {
                n140 = Send Notification(notification="postsweep", notifier=w361) -> ()  [unwired: 1 in, 2 out]
              }
            }
            n141 = local read "Center Frequency (Hz)"() -> (w332:dbl)
            n142 = local read "HW Channel"() -> (w276:i32)
            n143 = Subtract(x="Center Frequency (Hz)", y="Bandwidth (Hz)") -> (x-y=w281:dbl)
            n144 = Add(x="Center Frequency (Hz)", y="Bandwidth (Hz)") -> (x+y=w280:dbl)
            n145 = Index Array(array=w360, index (col)=0 ("disabled index (col)")) -> (element=w347:dbl[])  [unwired: 1 in]
            n146 = local write "fmax"(w280) -> ()
            n147 = local write "fmin"(w281) -> ()
            n148 = Equal To 0?(x=w276) -> (x = 0?=w275:bool)
            n149 = call <instrlib>:"ziBW2TC.vi"("Order (1)"=w288, "BW (Hz)"=w331) -> ("TC (s)"=w286:dbl)  [unwired: 1 in]
            n150 = local read "Sweep Oscillator"() -> (w308:i32)
            n151 = Subtract(x=w347, y=w332) -> (x-y=w287:dbl[])
            n152 = local read "Output Demod"() -> (w307:i32)
            n153 = Select(t=w279, s=w275, f=w278) -> (s? t:f=w277:i32)
            n154 = local read "Output Demod"() -> (w297:i32)
            n155 = Build Array(w277) -> (w330:i32[])
            n156 = Absolute Value(x=w287) -> (abs(x)=w290:dbl[])
            n157 = local read "HW Channel"() -> (w298:i32)
            n158 = call <instrlib>:"ziSweeper.vi"("Handle In"=w285, "Output Channel (6)"=w307, "Sweep Sequence"=w360, "Oscillator (0)"=w308, "Error In"=w284, "Input Demods (0)"=w330) -> ("Handle Out"=w302:T4, "Output (F,X1,Y1,X2,Y2,...,Vo)"=w359:dbl[][], "Error Out"=w301:errorcluster)  [unwired: 7 in]
            n159 = Compound Arithmetic op=MULTIPLY(cdb 0.0+2.0i ("r * e^(i*theta)"), 3.141592653589793, w286) -> (w294:cdb)
            n160 = Multiply(x=w294, y=w290) -> (x*y=w291:cdb[])
            n161 = Increment(x=w291) -> (x+1=w293:cdb[])
            n162 = local read "HW Channel"() -> (w271:i32)
            n163 = Format Into String(format string="sigouts/%u/amplitudes/%u" ("Cursor.Cursor Name"), w298, w297) -> (resulting string=w299:string)  [unwired: 2 in, 1 out]
            n164 = Reciprocal(x=w293) -> (1/x=w292:cdb[])
            n165 = Index Array(array=w359, index (col) #1=0 ("disabled index (col)"), index (col) #2=1 ("index (col)"), index (col) #3=2 ("index (col)")) -> (element #1=w324:dbl[], element #2=w358:dbl[], element #3=w357:dbl[])  [unwired: 3 in]
            n166 = Power Of X(1:w292, 2:w288) -> (0:w289:cdb[])
            n167 = call <instrlib>:"ziGetValueDouble.vi"("error in"=w301, "Path"=w299, "Handle in"=w302) -> ("error out"=w267:errorcluster, "Value"=w263:dbl, "Handle out"=w269:T4)
            n168 = Re/Im To Polar(2:w357, 3:w358) -> (0:w352:dbl[], 1:w304:dbl[])
            n169 = Complex To Polar(r * e^(i*theta)=w289) -> (r=w348:dbl[])  [unwired: 1 out]
            n170 = Format Into String(format string="sigouts/%u/range" ("Cursor.Cursor Name"), w271) -> (resulting string=w265:string)  [unwired: 2 in, 1 out]
            n171 = expression code="20*log(x)"(w348) -> (w349:dbl[])
            n172 = call <vilib>:"Unwrap Phase.vi"("phase unit"=w351, "Phase"=w352) -> ("Unwrapped Phase"=w321:dbl[])  [unwired: 8 in, 1 out]
            n173 = call <instrlib>:"ziGetValueDouble.vi"("error in"=w267, "Path"=w265, "Handle in"=w269) -> ("error out"=w266:errorcluster, "Value"=w262:dbl, "Handle out"=w268:T4)
            n174 = Multiply(x=w263, y=w262) -> (x*y=w264:dbl)
            n175 = Divide(x=w304, y=w264) -> (x/y=w303:dbl[])
            n176 = local read "Q Control"() -> (w317:bool)
            n177 = Initialize Array(cluster{dbl[], dbl[]} {[], []}, 2 ("dimension size")) -> (w312:cluster{dbl[], dbl[]}[])
            n178 = expression code="20*log(x)"(w303) -> (w353:dbl[])
            n179 = Rotate 1D Array(1:w324, 2:-1 ("n")) -> (0:w325:dbl[])
            n180 = Rotate 1D Array(1:w324, 2:1 ("n")) -> (0:w342:dbl[])
            n181 = Rotate 1D Array(1:w321, 2:-1 ("n")) -> (0:w322:dbl[])
            n182 = Rotate 1D Array(1:w321, 2:1 ("n")) -> (0:w343:dbl[])
            n183 = Select(t=1, s=w317, f=0 ("index")) -> (s? t:f=w310:i32)
            n184 = Bundle("Output (F,X1,Y1,X2,Y2,...,Vo)"=w324, w353) -> (w326:T8)  [unwired: 1 in]
            n185 = Bundle("Output (F,X1,Y1,X2,Y2,...,Vo)"=w324, "Unwrapped Phase"=w321) -> (w311:T9)  [unwired: 1 in]
            n186 = Bundle("Output (F,X1,Y1,X2,Y2,...,Vo)"=w324, w349) -> (w316:T8)  [unwired: 1 in]
            n187 = Subtract(x=w325, y=w342) -> (x-y=w339:dbl[])
            n188 = Subtract(x=w322, y=w343) -> (x-y=w340:dbl[])
            n189 = feedback #1(w312) -> (w314:cluster{dbl[], dbl[]}[])
            n190 = Divide(x=w340, y=w339) -> (x/y=w338:dbl[])
            n191 = Replace Array Subset(array=w314, new element=w326, index=w310) -> (w335:cluster{dbl[], dbl[]}[])
            n192 = feedback #2(w312) -> (w313:cluster{dbl[], dbl[]}[])
            n193 = Replace Array Subset(array=w313, new element=w311, index=w310) -> (w309:cluster{dbl[], dbl[]}[])
            n194 = Multiply(x=1.0 ("Timeconstant (s)"), y=w338) -> (x*y=w329:dbl[])
            n195 = Build Array(w324, w329) -> (w328:dbl[][])
            n196 = for {
              tunnel: w328 -> [w376] mode=indexing
              tunnel: [w371] -> w327 mode=indexing
              n197 = Delete From Array(array=w376, length=1, index=0) -> (array with subset deleted=w372:dbl[])  [unwired: 1 out]
              n198 = Array Size(array=w372) -> (size(s)=w374:i32)
              n199 = Decrement(x=w374) -> (x-1=w373:i32)
              n200 = Delete From Array(array=w372, length=1, index=w373) -> (array with subset deleted=w371:dbl[])  [unwired: 1 out]
            }
            n201 = Index Array(array=w327) -> (element #1=w272:dbl[], element #2=w273:dbl[])  [unwired: 4 in]
            n202 = Multiply(x=100.0 ("Timeconstant (s)"), y=w273) -> (x*y=w336:dbl[])
            n203 = Bundle(w272, w336) -> (w346:cluster{dbl[], dbl[]})  [unwired: 1 in]
            n204 = case shown="False" w305 {
              tunnel: w335 -> [w363 w366]
              tunnel: w316 -> [_ w365]
              tunnel: [w363 w364] -> w315
              frame #0 {
              }
              frame #1 {
                n205 = Build Array (concatenate)(w366, w365) -> (w364:T2)
              }
            }
            "Graph Amplitude" <- w315
            n206 = case shown="False" w305 {
              tunnel: w346 -> [_ w370]
              tunnel: [w367 w369] -> w345
              tunnel: w309 -> [w367 w368]
              frame #0 {
              }
              frame #1 {
                n207 = Build Array (concatenate)(w368, w370) -> (w369:cluster{dbl[], dbl[]}[])
              }
            }
            "Graph Phase" <- w345
          }
          frame #1 {
            # "derivatives"
            # "frequencies"
            n208 = local read "Q Control"() -> (w393:bool)
            n209 = flat-sequence {
              frame #0 {
                n210 = control-ref of="Tab Control QControl"() -> (w435:refnum<vi>)
                n211 = control-ref of="Tab Control Sweep"() -> (w434:refnum<vi>)
                n212 = property on="Run" class="Bool (strict)"("DisabledEnum"=T6."Enabled" ("Disabled"), "Value"=FALSE ("Run")) -> ()  [unwired: 2 in, 2 out]
                n213 = Build Array(w435, w434) -> (w430:refnum<vi>[])
                n214 = Index Array(array=w430) -> (element #1=w429:refnum<vi>)  [unwired: 2 in, 1 out]
                n215 = property class="TabCtl"(reference=w429) -> ("Pages"=w433:refnum<vi>[])  [unwired: 1 in, 2 out]
                n216 = Index Array(array=w433) -> (element #3=w431:refnum<vi>)  [unwired: 3 in, 2 out]
                n217 = property class="Page"(reference=w431, "PageEnb"=T5."Page Enabled" ("Page Enabled State")) -> ()  [unwired: 1 in, 2 out]
              }
            }
            n218 = Select(t=u32 1 ("Active Cursor"), s=w393, f=u32 0 ("Active Cursor")) -> (s? t:f=w394:u32)
            n219 = Index Array(array=w390, index (row)=w394) -> (element=w396:refnum<vi>[])  [unwired: 1 in]
            n220 = for {
              tunnel: w396 -> [w438] mode=indexing
              n221 = Not A Number/Path/Refnum?(number/path/refnum=w438) -> (NaN/Path/Refnum?=w439:bool)
              n222 = case shown="False" w439 {
                tunnel: w438 -> [w442 _]
                tunnel: T6."Enabled" ("Disabled") -> [w441 _]
                frame #0 {
                  n223 = property class="DigNum (strict)"(reference=w442, "DisabledEnum"=w441) -> ()  [unwired: 1 in, 2 out]
                }
                frame #1 {
                }
              }
            }
            n224 = local read "Q Control"() -> (w398:bool)
            n225 = Array Max & Min(array=w391) -> (min value=w412:dbl, min index (indices)=w417:i32)  [unwired: 2 out]
            n226 = local read "AutoCenter"() -> (w387:bool)
            n227 = Index Array(array=w392, index=w417) -> (element=w404:dbl)
            n228 = Select(t=u32 1 ("Active Cursor"), s=w398, f=u32 0 ("Active Cursor")) -> (s? t:f=w402:u32)
            n229 = case shown="True" w387 {
              frame #0 {
              }
              frame #1 {
                n230 = local read "Resonance Freq (Hz)"() -> (w428:dbl)
                n231 = control-ref of="Center Frequency (Hz)"() -> (w427:refnum<vi>)
                n232 = property class="DigNum (strict)"(reference=w427, "Val(Sgnl)"=w428) -> ()  [unwired: 1 in, 2 out]
              }
            }
            n233 = Divide(x=6.283185307179586, y=360.0 ("value")) -> (x/y=w413:dbl)
            n234 = Compound Arithmetic op=MULTIPLY(w413, w404, w412, -0.5 ("value")) -> (w400:dbl)
            n235 = disable-structure shown="Disabled" {
              disable-tunnel: [w423 "controlled" ("Cursor.Cursor Name")] -> w401
              disable-tunnel: w400 -> [w421 _]
              disable-tunnel: [w420 "native" ("Cursor.Cursor Name")] -> w399
              frame #0 {
                n236 = Format Into String(format string="controlled\nQ=%f" ("Cursor.Cursor Name"), w421) -> (resulting string=w423:string)  [unwired: 2 in, 1 out]
                n237 = Format Into String(format string="native\nQ=%f" ("Cursor.Cursor Name"), w421) -> (resulting string=w420:string)  [unwired: 2 in, 1 out]
              }
              frame #1 {
              }
            }
            n238 = Select(t=w401, s=w398, f=w399) -> (s? t:f=w410:string)
            n239 = for {
              tunnel: w397 -> [w451] mode=indexing
              tunnel: w402 -> [w443]
              tunnel: w404 -> [w450]
              tunnel: w410 -> [w449]
              tunnel: [w448] -> w409 mode=indexing
              n240 = property class="XYGraph (strict)"(reference=w451, "Active Cursor"=w443, "Cursor.Visible"=TRUE, "Cursor.Cursor X"=w450, "Cursor.Cursor Name"=w449, "Cursor.Cursor Name Visible"=TRUE ("Cursor Legend Visible"), "Cursor.Cursor Color"=u32 16771584, "Cursor.Cursor Style"=u8 1, "Cursor.Cursor Plot"=w443) -> ("Cursor.Cursor Y"=w448:dbl)  [unwired: 1 in, 2 out]
            }
            n241 = Index Array(array=w409) -> (element #1=w407:dbl, element #2=w408:dbl)  [unwired: 2 in]
            n242 = Multiply(x=2, y=w400) -> (x*y=w405:dbl)
            n243 = Divide(x=w404, y=w405) -> (x/y=w403:dbl)
            n244 = case shown="False" w398 {
              tunnel: w404 -> [w459 w462]
              tunnel: w400 -> [w460 w463]
              tunnel: w408 -> [w456 _]
              tunnel: w407 -> [w457 _]
              tunnel: w403 -> [w452 w461]
              frame #0 {
                w455 = T6."Enabled" ("Disabled")
                n245 = property on="Q Enhancement" class="Slide (strict)"() -> ("Value"=w453:dbl)  [unwired: 2 in, 2 out]
                n246 = property on="f/2Q (Hz)" class="DigNum (strict)"("Val(Sgnl)"=w452) -> ()  [unwired: 2 in, 2 out]
                n247 = control-ref of="Phase Shift (°)"() -> (w458:refnum<vi>)
                n248 = property on="Resonance Freq (Hz)" class="DigNum (strict)"("Val(Sgnl)"=w459) -> ()  [unwired: 2 in, 2 out]
                n249 = property class="DigNum (strict)"(reference=w458, "Val(Sgnl)"=w456) -> ()  [unwired: 1 in, 2 out]
                n250 = property on="PID Drive Limit (V)" class="DigNum (strict)"("DisabledEnum"=T6."Enabled" ("Disabled")) -> ()  [unwired: 2 in, 2 out]
                n251 = property on="Q Enhancement" class="Slide (strict)"("Val(Sgnl)"=w453) -> ()  [unwired: 2 in, 2 out]
                n252 = property on="Q Enhancement" class="Slide (strict)"("DisabledEnum"=w455) -> ()  [unwired: 2 in, 2 out]
                n253 = property on="Q Control" class="Bool (strict)"("DisabledEnum"=w455) -> ()  [unwired: 2 in, 2 out]
                "Q Factor" <- w460
                "Gain Margin (dB)" <- w457
              }
              frame #1 {
                n254 = property on="Characteristic Frequency Q" class="DigNum (strict)"("Val(Sgnl)"=w461) -> ()  [unwired: 2 in, 2 out]
                "controlled" <- w463
                "Resonance Frequency Q" <- w462
              }
            }
            n255 = property on="Graph Phase" class="XYGraph (strict)"("DisabledEnum"=T6."Enabled" ("Disabled")) -> ()  [unwired: 2 in, 2 out]
            n256 = property on="Graph Amplitude" class="XYGraph (strict)"("DisabledEnum"=T6."Enabled" ("Disabled")) -> ()  [unwired: 2 in, 2 out]
          }
        }
      }
    }
    n257 = local read "stop"() -> (w65:bool)
  }
  n258 = while {
    shift-right: [w468] -> w40
    shift-left: w41 -> [w469]
    shift-right: [w466] -> w38
    shift-left: w39 -> [w467]
    tunnel: w37 -> [w465]
    tunnel: w9 -> [w464]
    stop <- w471 stop-if-true
    n259 = event shown="[1] Panel Close;  Application Instance Close" {
      selector: _ -> [_ _ _ _ _ _ _ _ _ _ _ _ _ _ _ _ _ _ _ _ _]
      dyn-events: _ -> [_ _ _ _ _ _ _ _ _ _ _ _ _ _ _ _ _ _ _ _ _]
      timeout: 50 -> [_ _ _ _ _ _ _ _ _ _ _ _ _ _ _ _ _ _ _ _ _]
      tunnel: w469 -> [w473 w476 w486 w496 w514 w529 w559 w572 w594 w596 w603 w608 w612 w621 w625 w642 w646 w659 w686 w703 w732]
      tunnel: [w473 w476 w483 w493 w521 w545 w559 w572 w594 w596 w603 w608 w612 w621 w625 w642 w646 w659 w685 w702 w731] -> w468
      tunnel: w467 -> [w472 w475 w485 w495 w511 w526 w558 w571 w593 w595 w602 w607 w611 w620 w624 w641 w645 w658 w683 w700 w729]
      tunnel: [w472 w475 w482 w492 w520 w544 w558 w571 w593 w595 w602 w607 w611 w620 w624 w641 w645 w658 w684 w701 w730] -> w466
      tunnel: w465 -> [_ _ _ _ _ _ _ _ w591 w597 _ _ _ _ _ _ _ _ _ _ _]
      tunnel: w464 -> [_ _ _ _ _ _ _ _ _ _ _ _ _ _ w627 _ _ _ _ _ _]
      event #0 {
        n260 = event-data() -> ()  [unwired: 1 in, 2 out]
      }
      event #1 {
        n261 = event-data() -> ()  [unwired: 1 in, 2 out]
        n262 = local write "stop"(TRUE ("stop")) -> ()
      }
      event #2 {
        n263 = event-data() -> ("NewVal"=w484:dbl)  [unwired: 1 in, 4 out]
        n264 = local read "HW Channel"() -> (w478:i32)
        n265 = Equal To 0?(x=w478) -> (x = 0?=w477:bool)
        n266 = Select(t="demods/0/phaseshift" ("Path"), s=w477, f="demods/3/phaseshift") -> (s? t:f=w479:string)
        n267 = call-poly <instrlib>:"ziSetValue.vi"("Error In"=w485, "Value"=w484, "Path"=w479, "Handle In"=w486) -> ("Error Out"=w482:errorcluster, "Handle Out"=w483:T4)  [unwired: 1 in]
      }
      event #3 {
        n268 = event-data() -> ("NewVal"=w494:dbl)  [unwired: 1 in, 4 out]
        n269 = local read "PIDs"() -> (w487:i32)
        n270 = Index Array(array=dbl[][] [[0.0, 1.0], [2.0, 3.0]], index (row)=w487) -> (element=w489:dbl[])  [unwired: 1 in]
        n271 = for {
          tunnel: "pids/%u/range" ("Path") -> [w505]
          tunnel: w489 -> [w504] mode=indexing
          tunnel: [w503] -> w488 mode=indexing
          n272 = Format Into String(format string=w505, w504) -> (resulting string=w503:string)  [unwired: 2 in, 1 out]
        }
        n273 = for {
          tunnel: w494 -> [w500]
          shift-right: [w499] -> w493
          shift-left: w496 -> [w502]
          tunnel: w488 -> [w497] mode=indexing
          shift-right: [w498] -> w492
          shift-left: w495 -> [w501]
          n274 = call-poly <instrlib>:"ziSetValue.vi"("Error In"=w501, "Value"=w500, "Path"=w497, "Handle In"=w502) -> ("Error Out"=w498:errorcluster, "Handle Out"=w499:T4)  [unwired: 1 in]
        }
      }
      event #4 {
        n275 = event-data() -> ("NewVal"=w508:dbl)  [unwired: 1 in, 4 out]
        n276 = local read "Output Demod"() -> (w517:i32)
        n277 = local read "HW Channel"() -> (w516:i32)
        n278 = local read "HW Channel"() -> (w518:i32)
        n279 = Format Into String(format string="sigouts/%u/amplitudes/%u" ("Cursor.Cursor Name"), w516, w517) -> (resulting string=w506:string)  [unwired: 2 in, 1 out]
        n280 = Format Into String(format string="sigouts/%u/range" ("Cursor.Cursor Name"), w518) -> (resulting string=w510:string)  [unwired: 2 in, 1 out]
        n281 = call <instrlib>:"ziGetValueDouble.vi"("error in"=w511, "Path"=w510, "Handle in"=w514) -> ("error out"=w512:errorcluster, "Value"=w509:dbl, "Handle out"=w513:T4)
        n282 = Divide(x=w508, y=w509) -> (x/y=w507:dbl)
        n283 = call-poly <instrlib>:"ziSetValue.vi"("Error In"=w512, "Value"=w507, "Path"=w506, "Handle In"=w513) -> ("Error Out"=w520:errorcluster, "Handle Out"=w521:T4)  [unwired: 1 in]
      }
      event #5 {
        n284 = event-data() -> ()  [unwired: 1 in, 5 out]
        n285 = local read "Oscillator"() -> (w523:i32)
        n286 = local read "Center Frequency (Hz)"() -> (w525:dbl)
        n287 = Format Into String(format string="oscs/%u/freq", w523) -> (resulting string=w522:string)  [unwired: 2 in, 1 out]
        n288 = local read "HW Channel"() -> (w538:i32)
        n289 = local read "Bandwidth (Hz)"() -> (w539:dbl)
        n290 = call-poly <instrlib>:"ziSetValue.vi"("Error In"=w526, "Value"=w525, "Path"=w522, "Handle In"=w529) -> ("Error Out"=w527:errorcluster, "Handle Out"=w528:T4)  [unwired: 1 in]
        n291 = Equal To 0?(x=w538) -> (x = 0?=w534:bool)
        n292 = Select(t=string[] ["demods/0/timeconstant"], s=w534, f=string[] ["demods/4/timeconstant"]) -> (s? t:f=w535:string[])
        n293 = call <instrlib>:"ziBW2TC.vi"("Order (1)"=4 ("Order (#)"), "BW (Hz)"=w539) -> ("TC (s)"=w530:dbl)  [unwired: 1 in]
        n294 = for {
          shift-right: [w549] -> w542
          shift-left: w528 -> [w551]
          shift-right: [w548] -> w541
          shift-left: w527 -> [w550]
          tunnel: w530 -> [w547]
          tunnel: w535 -> [w546] mode=indexing
          n295 = call-poly <instrlib>:"ziSetValue.vi"("Error In"=w550, "Value"=w547, "Path"=w546, "Handle In"=w551) -> ("Error Out"=w548:errorcluster, "Handle Out"=w549:T4)  [unwired: 1 in]
        }
        n296 = Select(t=string[] ["demods/0/oscselect", "demods/1/oscselect", "demods/2/oscselect"], s=w534, f=string[] ["demods/3/oscselect", "demods/4/oscselect", "demods/5/oscselect"]) -> (s? t:f=w531:string[])
        n297 = for {
          shift-right: [w555] -> w545
          shift-left: w542 -> [w557]
          shift-right: [w554] -> w544
          shift-left: w541 -> [w556]
          tunnel: "Oscillator" -> [w553]
          tunnel: w531 -> [w552] mode=indexing
          n298 = call-poly <instrlib>:"ziSetValue.vi"("Error In"=w556, "Value"=w553, "Path"=w552, "Handle In"=w557) -> ("Error Out"=w554:errorcluster, "Handle Out"=w555:T4)  [unwired: 1 in]
        }
      }
      event #6 {
        n299 = event-data() -> ()  [unwired: 1 in, 5 out]
        n300 = disable-structure shown="Disabled" {
          frame #0 {
            n301 = local read "Characteristic Frequency Q"() -> (w565:dbl)
            n302 = local read "f/2Q (Hz)"() -> (w564:dbl)
            n303 = local read "Q Control"() -> (w566:bool)
            n304 = Select(t=w565, s=w566, f=w564) -> (s? t:f=w563:dbl)
            n305 = Multiply(x=0.3, y=w563) -> (x*y=w562:dbl)
            n306 = local read "AutoBW"() -> (w560:bool)
            n307 = case shown="True" w560 {
              tunnel: [T6."Enabled" ("Disabled") T6."Disabled and Grayed Out" ("Disabled")] -> w567
              tunnel: w562 -> [_ w569]
              frame #0 {
              }
              frame #1 {
                n308 = local write "BW (Hz)"(w569) -> ()
              }
            }
            n309 = property on="BW (Hz)" class="DigNum (strict)"("DisabledEnum"=w567) -> ()  [unwired: 2 in, 2 out]
          }
          frame #1 {
          }
        }
      }
      event #7 {
        n310 = event-data() -> ("NewVal"=w578:dbl)  [unwired: 1 in, 4 out]
        n311 = local read "Gain Margin (dB)"() -> (w582:dbl)
        n312 = Less?(x=w578, y=1.0) -> (x < y?=w574:bool)
        n313 = Reciprocal(x=w578) -> (1/x=w579:dbl)
        n314 = expression code="10**(x/20)"(w582) -> (w581:dbl)
        n315 = Subtract(x=1.0, y=w579) -> (x-y=w580:dbl)
        n316 = Divide(x=w580, y=w581) -> (x/y=w576:dbl)
        n317 = case shown="True" w574 {
          tunnel: w576 -> [w586 w589]
          tunnel: [w586 w588] -> w573
          tunnel: [FALSE ("Invert Gain") TRUE ("Invert Gain")] -> w575
          frame #0 {
          }
          frame #1 {
            n318 = Negate(x=w589) -> (-x=w588:dbl)
          }
        }
        n319 = flat-sequence {
          tunnel: w575 -> [w584]
          tunnel: w573 -> [w585]
          frame #0 {
            n320 = property on="Invert Gain" class="Bool (strict)"("Value"=w584) -> ()  [unwired: 2 in, 2 out]
          }
          frame #1 {
            n321 = property on="Feedback Gain (V/Vrms)" class="Slide (strict)"("Val(Sgnl)"=w585) -> ()  [unwired: 2 in, 2 out]
          }
        }
      }
      event #8 {
        n322 = event-data() -> ()  [unwired: 1 in, 5 out]
        n323 = Send Notification(notification="setup", notifier=w591) -> ()  [unwired: 1 in, 2 out]
      }
      event #9 {
        n324 = event-data() -> ()  [unwired: 1 in, 5 out]
        n325 = Send Notification(notification="sweep", notifier=w597) -> ()  [unwired: 1 in, 2 out]
      }
      event #10 {
        n326 = event-data() -> ("NewVal"=w600:dbl)  [unwired: 1 in, 4 out]
        n327 = local read "AutoCenter"() -> (w599:bool)
        n328 = case shown="True" w599 {
          tunnel: w600 -> [_ w604]
          frame #0 {
          }
          frame #1 {
            n329 = local write "Center Frequency (Hz)"(w604) -> ()
          }
        }
        n330 = property on="AutoCenter" class="Bool (strict)"("DisabledEnum"=T6."Enabled" ("Disabled")) -> ()  [unwired: 2 in, 2 out]
      }
      event #11 {
        n331 = event-data() -> ("NewVal"=w606:dbl)  [unwired: 1 in, 4 out]
        n332 = local read "AutoPhase"() -> (w605:bool)
        n333 = case shown="True" w605 {
          tunnel: w606 -> [_ w610]
          frame #0 {
          }
          frame #1 {
            n334 = Negate(x=w610) -> (-x=w609:dbl)
            n335 = property on="Feedback Phase (deg)" class="Slide (strict)"("Val(Sgnl)"=w609) -> ()  [unwired: 2 in, 2 out]
          }
        }
      }
      event #12 {
        n336 = event-data() -> ("NewVal"=w613:bool)  [unwired: 1 in, 4 out]
        n337 = case shown="True" w613 {
          frame #0 {
          }
          frame #1 {
            n338 = local read "Resonance Freq (Hz)"() -> (w614:dbl)
            n339 = local write "Center Frequency (Hz)"(w614) -> ()
          }
        }
      }
      event #13 {
        n340 = event-data() -> ("NewVal"=w616:bool)  [unwired: 1 in, 4 out]
        n341 = case shown="True" w616 {
          frame #0 {
          }
          frame #1 {
            n342 = local read "Phase Shift (°)"() -> (w622:dbl)
            n343 = Negate(x=w622) -> (-x=w623:dbl)
            n344 = property on="Feedback Phase (deg)" class="Slide (strict)"("Val(Sgnl)"=w623) -> ()  [unwired: 2 in, 2 out]
          }
        }
        n345 = control-ref of="Feedback Phase (deg)"() -> (w615:refnum<vi>)
        n346 = Select(t=T6."Disabled and Grayed Out" ("Disabled"), s=w616, f=T6."Enabled" ("Disabled")) -> (s? t:f=w619:T6)
        n347 = property class="Slide (strict)"(reference=w615, "DisabledEnum"=w619) -> ()  [unwired: 1 in, 2 out]
      }
      event #14 {
        n348 = event-data() -> ("NewVal"=w626:bool)  [unwired: 1 in, 4 out]
        n349 = for {
          tunnel: w627 -> [w631] mode=indexing
          tunnel: w626 -> [w629]
          n350 = property class="XYGraph (strict)"(reference=w631, "Active Plot"=u32 2, "Plot.Visible?"=w629) -> (error out=w628:errorcluster)  [unwired: 1 in, 1 out]
          n351 = call <vilib>:"Clear Errors.vi"("error in (no error)"=w628) -> ()  [unwired: 6 in, 1 out]
        }
      }
      event #15 {
        n352 = event-data() -> ("NewVal"=w634:bool)  [unwired: 1 in, 4 out]
        n353 = control-ref of="ADC Over"() -> (w632:refnum<vi>)
        n354 = control-ref of="Stability Warning"() -> (w633:refnum<vi>)
        n355 = control-ref of="Invert Gain"() -> (w640:refnum<vi>)
        n356 = control-ref of="Feedback Gain (V/Vrms)"() -> (w639:refnum<vi>)
        n357 = Build Array(w632, w633, w640, w639) -> (w638:refnum<vi>[])
        n358 = Select(t=T6."Disabled and Grayed Out" ("Disabled"), s=w634, f=T6."Enabled" ("Disabled")) -> (s? t:f=w637:T6)
        n359 = for {
          tunnel: w638 -> [w644] mode=indexing
          tunnel: w637 -> [w643]
          n360 = property class="Ctl"(reference=w644, "DisabledEnum"=w643) -> ()  [unwired: 1 in, 2 out]
        }
      }
      event #16 {
        n361 = event-data() -> ("CtlRef"=w650:refnum<vi>, "NewVal"=w649:dbl)  [unwired: 1 in, 3 out]
        n362 = local read "BW (Hz)"() -> (w648:dbl)
        n363 = Less?(x=w649, y=w648) -> (x < y?=w647:bool)
        n364 = property class="DigNum (strict)"(reference=w650, "Blinking"=w647) -> ()  [unwired: 1 in, 2 out]
      }
      event #17 {
        n365 = event-data() -> ("CtlRef"=w660:refnum<vi>, "NewVal"=w655:dbl)  [unwired: 1 in, 3 out]
        n366 = control-ref of="f/2Q (Hz)"() -> (w654:refnum<vi>)
        n367 = control-ref of="Characteristic Frequency Q"() -> (w653:refnum<vi>)
        n368 = Build Array(w654, w653) -> (w651:refnum<vi>[])
        n369 = for {
          shift-right: [w671] -> w656
          shift-left: FALSE ("x > y?") -> [w670]
          tunnel: w655 -> [w668]
          tunnel: [w666] -> w652 mode=indexing
          tunnel: w651 -> [w663] mode=indexing
          n370 = property class="DigNum (strict)"(reference=w663) -> ("DisabledEnum"=w665:T6, "Value"=w664:dbl)  [unwired: 1 in, 2 out]
          n371 = Less?(x=w664, y=w668) -> (x < y?=w667:bool)
          n372 = Equal?(x=T6."Enabled" ("DisabledEnum"), y=w665) -> (x = y?=w669:bool)
          n373 = And(x=w669, y=w667) -> (x .and. y?=w666:bool)
          n374 = Or(x=w666, y=w670) -> (x .or. y?=w671:bool)
        }
        n375 = property class="DigNum (strict)"(reference=w660, "Blinking"=w656) -> ()  [unwired: 1 in, 2 out]
        n376 = for {
          tunnel: w652 -> [w662] mode=indexing
          tunnel: w651 -> [w661] mode=indexing
          n377 = property class="DigNum (strict)"(reference=w661, "Blinking"=w662) -> ()  [unwired: 1 in, 2 out]
        }
      }
      event #18 {
        n378 = event-data() -> ("NewVal"=w675:i32)  [unwired: 1 in, 4 out]
        n379 = local read "Input Demod"() -> (w674:i32)
        n380 = local read "HW Channel"() -> (w673:i32)
        n381 = Format Into String(format string="demods/%u/adcselect", w674) -> (resulting string=w680:string)  [unwired: 2 in, 1 out]
        n382 = Format Into String(format string="demods/%u/oscselect", w674) -> (resulting string=w679:string)  [unwired: 2 in, 1 out]
        n383 = Bundle(w679, "NewVal"=w675) -> (w678:cluster{string, "NewVal":i32})  [unwired: 1 in]
        n384 = Bundle(w680, "HW Channel"=w673) -> (w677:cluster{string, "HW Channel":i32})  [unwired: 1 in]
        n385 = Build Array(w677, w678) -> (w676:cluster{string, "NewVal":i32}[])
        n386 = for {
          tunnel: w686 -> [w693]
          tunnel: [w690] -> w685
          tunnel: [w692] -> w684
          tunnel: w683 -> [w691]
          tunnel: w676 -> [w689] mode=indexing
          n387 = Unbundle(w689) -> (w688:string, "NewVal"=w687:i32)
          n388 = call-poly <instrlib>:"ziSetValue.vi"("Error In"=w691, "Value"=w687, "Path"=w688, "Handle In"=w693) -> ("Error Out"=w692:errorcluster, "Handle Out"=w690:T4)  [unwired: 1 in]
        }
      }
      event #19 {
        n389 = event-data() -> ("NewVal"=w694:bool)  [unwired: 1 in, 4 out]
        n390 = local read "HW Channel"() -> (w695:i32)
        n391 = Equal To 0?(x=w695) -> (x = 0?=w696:bool)
        n392 = Boolean To (0,1)(Boolean=w694) -> (0, 1=w704:i16)
        n393 = Select(t=string[] ["sigouts/0/enables/1", "sigouts/0/enables/2"], s=w696, f=string[] ["sigouts/1/enables/4", "sigouts/1/enables/5"]) -> (s? t:f=w699:string[])
        n394 = for {
          tunnel: w704 -> [w710]
          tunnel: w699 -> [w709] mode=indexing
          tunnel: w703 -> [w708]
          tunnel: [w707] -> w702
          tunnel: [w706] -> w701
          tunnel: w700 -> [w705]
          n395 = call-poly <instrlib>:"ziSetValue.vi"("Error In"=w705, "Value"=w710, "Path"=w709, "Handle In"=w708) -> ("Error Out"=w706:errorcluster, "Handle Out"=w707:T4)  [unwired: 1 in]
        }
      }
      event #20 {
        n396 = event-data() -> ("NewVal"=w722:dbl)  [unwired: 1 in, 4 out]
        n397 = local read "Gain Margin (dB)"() -> (w726:dbl)
        n398 = local read "PIDs"() -> (w712:i32)
        n399 = Negate(x=w722) -> (-x=w723:dbl)
        n400 = Index Array(array=dbl[][] [[0.0, 1.0], [2.0, 3.0]], index (row)=w712) -> (element=w713:dbl[])  [unwired: 1 in]
        n401 = Select(t=w723, s="Invert Gain", f=w722) -> (s? t:f=w721:dbl)
        n402 = expression code="10**(x/20)"(w726) -> (w725:dbl)
        n403 = for {
          tunnel: "pids/%u/P" -> [w735]
          tunnel: w713 -> [w734] mode=indexing
          tunnel: [w733] -> w711 mode=indexing
          n404 = Format Into String(format string=w735, w734) -> (resulting string=w733:string)  [unwired: 2 in, 1 out]
        }
        n405 = Multiply(x=w725, y=w721) -> (x*y=w724:dbl)
        n406 = Subtract(x=1.0, y=w724) -> (x-y=w720:dbl)
        n407 = Reciprocal(x=w720) -> (1/x=w717:dbl)
        n408 = Less Than 0?(x=w720) -> (x < 0?=w719:bool)
        "Stability Warning" <- w719
        n409 = for {
          tunnel: w732 -> [w741]
          tunnel: [w740] -> w731
          tunnel: [w739] -> w730
          tunnel: w729 -> [w738]
          tunnel: w721 -> [w737]
          tunnel: w711 -> [w736] mode=indexing
          n410 = call-poly <instrlib>:"ziSetValue.vi"("Error In"=w738, "Value"=w737, "Path"=w736, "Handle In"=w741) -> ("Error Out"=w739:errorcluster, "Handle Out"=w740:T4)  [unwired: 1 in]
        }
        n411 = Select(t=inf, s=w719, f=w717) -> (s? t:f=w718:dbl)
        n412 = property on="Q Enhancement" class="Slide (strict)"("Value"=w718) -> ()  [unwired: 2 in, 2 out]
      }
    }
    n413 = local read "stop"() -> (w471:bool)
  }
  n414 = while {
    shift-right: [w755] -> w36
    shift-left: w5 -> [w757]
    shift-right: [w754] -> w35
    shift-left: w4 -> [w756]
    stop <- w758 stop-if-true
    n415 = call <instrlib>:"ziPollDataEx.vi"("error in"=w756, "Timeout ms (50)"=50 ("TimeOut ms (50)"), "Handle In"=w757) -> ("error out"=w754:errorcluster, "PathArray"=w751:string[], "Handle Out"=w755:T4, "Value Double"=w743:dbl, "Timed Out"=w748:bool, "Value Int"=w742:i32)  [unwired: 1 in, 2 out]
    n416 = Index Array(array=w751, index #1=1 ("index")) -> (element #1=w745:string, element #2=w744:string)  [unwired: 1 in]
    n417 = local read "HW Channel"() -> (w750:i32)
    n418 = Not(x=w748) -> (.not. x?=w747:bool)
    n419 = Decimal String To Number(string=w744) -> (number=w749:i32)  [unwired: 2 in, 1 out]
    n420 = Equal?(x=w749, y=w750) -> (x = y?=w746:bool)
    n421 = case shown="True" w747 {
      tunnel: w743 -> [_ w762]
      tunnel: w746 -> [_ w761]
      tunnel: w745 -> [_ w760]
      tunnel: w742 -> [_ w759]
      frame #0 {
      }
      frame #1 {
        n422 = case shown="\"STATUS\"" w760 {
          tunnel: w762 -> [_ _ w766]
          tunnel: w761 -> [_ _ w765]
          tunnel: w759 -> [w763 _ _]
          frame #0 {
            n423 = Not Equal To 0?(x=w763) -> (x != 0?=→"ADC Over":bool)
          }
          frame #1 {
          }
          frame #2 {
            n424 = case shown="True" w765 {
              tunnel: w766 -> [_ w767]
              frame #0 {
              }
              frame #1 {
                w774 = 1.0 ("upper limit")
                n425 = local read "fmax"() -> (w769:dbl)
                n426 = local read "fmin"() -> (w768:dbl)
                n427 = Subtract(x=w767, y=w768) -> (x-y=w776:dbl)
                n428 = Subtract(x=w769, y=w768) -> (x-y=w777:dbl)
                n429 = Divide(x=w776, y=w777) -> (x/y=w773:dbl)
                n430 = Equal?(x=w773, y=w774) -> (x = y?=w770:bool)
                n431 = In Range and Coerce(upper limit=w774, x=w773, lower limit=0.0) -> (In Range?=w771:bool)  [unwired: 1 out]
                n432 = Or(x=w770, y=w771) -> (x .or. y?=w772:bool)
                n433 = case shown="True" w772 {
                  tunnel: w773 -> [_ w778]
                  frame #0 {
                  }
                  frame #1 {
                    n434 = local write "Sweep Progress"(w778) -> ()
                  }
                }
              }
            }
          }
        }
      }
    }
    n435 = local read "stop"() -> (w758:bool)
  }
  n436 = call <instrlib>:"ziClose.vi"("Error In"=w38, "Handle In"=w40) -> ("Error Out"=w2:errorcluster)  [unwired: 2 in, 1 out]
  n437 = call <instrlib>:"ziClose.vi"("Error In"=w35, "Handle In"=w36) -> ("Error Out"=w1:errorcluster)  [unwired: 2 in, 1 out]
  n438 = case shown="True" "restore settings" {
    tunnel: w15 -> [_ w785]
    tunnel: w14 -> [w780 w784]
    tunnel: w13 -> [w779 w783]
    tunnel: [w780 w782] -> w12
    tunnel: [w779 w781] -> w11
    frame #0 {
    }
    frame #1 {
      n439 = call <instrlib>:"ziLoadSettings.vi"("Error in"=w783, "File path (dialog if empty)"=w785, "Handle in"=w784) -> ("Error out"=w781:errorcluster, "Handle out"=w782:T4)  [unwired: 2 in]
    }
  }
  n440 = call <instrlib>:"ziClose.vi"("Error In"=w11, "Handle In"=w12) -> ("Error Out"=w3:errorcluster)  [unwired: 2 in, 1 out]
  n441 = flat-sequence "Quit if running in compiled form" {
    tunnel: w3 -> [_]
    tunnel: w2 -> [_]
    tunnel: w1 -> [_]
    frame #0 {
      n442 = property class="App"() -> ("App.Kind"=w789:T10)  [unwired: 2 in, 2 out]
      n443 = local write "stop"(FALSE ("stop")) -> ()
      n444 = Equal?(x=w789, y=T10."Run Time System" ("Application:Kind")) -> (x = y?=w787:bool)
      n445 = Quit LabVIEW(quit? (T)=w787) -> ()
    }
  }
